vi "Preset_Manager_Main.vi"(4 "Virtual Devices List":string[](array[string]), 6 "Filtered Devices List":string[](array[string]), 8 "Experiment Name":string, 10 "DevStatusQueue":refnum<queue>, 11 "Software Root":string) -> ()   [LabVIEW 2020]
uses:
  Control 1.ctl
  <vilib>/Utility/miscctls.llb/LVRowAndColumnTypeDef.ctl
  Shared/MySQL/Preset Query Enum.ctl
  202ec612-3c63-4871-a0f5-fb571a4f3b4f.vi
  <vilib>/Array/Sort 2D Array - Pop Stack.vi
  <vilib>/Array/Sort 2D Array - Push Stack.vi
  <vilib>/Platform/browser.llb/Open URL in Default Browser (string).vi
  <vilib>/Utility/file.llb/Read Delimited Spreadsheet (string).vi
  <vilib>/Utility/file.llb/Write Delimited Spreadsheet (string).vi
  <userlib>/_OpenG.lib/array/array.llb/Delete Elements from 1D Array (String)__ogtk.vi
  <userlib>/_OpenG.lib/array/array.llb/Empty 1D Array (String)__ogtk.vi
  <vilib>/regexp/Match Regular Expression.xnode
panel:
  out "Queue Progress Bar":ext(slide) scale=0.0..1.0
  out "Queue Size":i32
  out "Current Preset Queue Element":string
  in  "Preset Devices Not On":i32(listbox)
  in  "Preset Devices Not in Experiment":i32(listbox)
  out "Active Preset":string
  out "Preset Execution Indicator":bool caption="Preset Aborted"
  in  "EXIT":bool
  in  "Using Queue":bool
  in  "Tab Control":T1(tab)
  in  "Dont jump \nto diagnostics":bool
  out "Currently Loaded":string
  in  "Reload Preset":bool caption="Reload"
  in  "Reload ECS":bool caption="Reload"
  in  "Preset Builder":bool
  in  "Execute Preset":bool
  in  "Delete Preset":bool
  in  "Save as Preset":bool
  in  "Preset Menu":u16(ring) items=["None", "2BL Amp2 16 J  Atte 100% BS 100T", "2BL Amp2 16 J Clunker IN 5% Attenuator", "2BL Amp2 16J Clunker OUT 5% att", "2BL Amp2 50/50", "2BL amp3 25 J 100T ", "2BL cameras triggered", "Amp 2 18 J 1BL", "Amp 3 25 J staging", "Amp2 Clunker In 1BL", "Amp2, MegaAttenuator", "Cameras free run - BELLA", "Cameras free run - DataLogging", "Cameras triggered - BELLA", "Cameras triggered - DataLogging", "Cameras triggered-1BL BELLA", "LT Amp1", "LT Amp2 17J", "LT Amp2 17J Clunker in", "LT Amp3 25 J Megaattenuator", "LT Amp3 25J", "LT Amp3 50J", "MagSpec TriggerOn", "MagSpecSimulateBoff", "MagSpecSimulateBon", "P2-WFS-LC", "SingleShot", "Stage 1 Cap in", "Stage 1 Cap out", "Stage 1 SMF in", "Stage 2 Gasjet IN", "Stage 2 Gasjet OUT", "Stage 2 SMF IN", "Stage 2 Tape Drive In and Aligned", "Stage 2 Tapedrive IN", "Stage 2 Tapedrive OUT", "Stage 2 YAG IN", "Staging APL In", "Staging APL out", "Z 1Hz", "Z Amp2 18 J", "Z Amp3 45 J 1BL Only", "Z Amp3 45 J OFI", "Z Amp3 45 J, Megaattenuator", "Z Diode obsolete", "Z amp2 , Clunker In", "Z amp2 12 J 80/20 OFI", "Z-Test-IN", "Z-Test22", "Z_TestPreset", "extra 2BL amp2 100T "]
  in  "Select an ECS file":path
  in  "Preset Table Control":string[][](table)
  in  "Choose Values":bool
  in  "Left Join":bool
  in  "Reset Queue":bool
  in  "Queue Table Control":string[][](table)
  in  "Queue Table":string[][](table)
  in  "Execute Queue":bool
  in  "Load Preset Queue":bool
  in  "Save Preset Queue":bool
  in  "Preset Queue Path":path
  out "Active Preset Achieved":bool
  out "Devices with Active \nPreset Not Set":string[](array[string])
  out "Dev Presets":string[](array[string])
  out "All Preset Devices ON?":bool[](array[boolean])
  in  "Abort Execution":T2
  in  "HELP WEB PAGE":bool
  out "PRESET FROM DB":string[][](table)
  out "ECS File":string[][](table)
  out "Coordinate Array":i32[][](array[numeric])
  out "Devices not started":string[](array[string]) caption="Devices not ready for scan"
  out "Active Device array":bool[](array[boolean])
  out "Active Dev/IP":string[](array[string])
  out "Device Errors":string[][](array[string])
  out "Queue Element":i32
  in  "Poll Count":i32
  out "error out":errorcluster
  out "Current State":string
  out "Remaining States":string
  # "Using CSV Files"
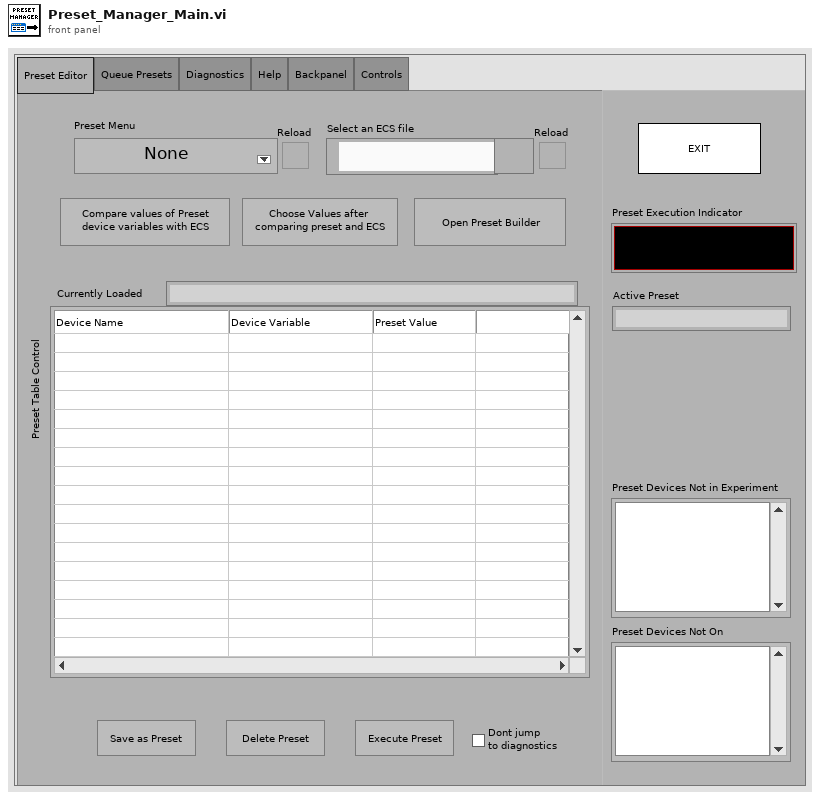
[diagram p1: front panel]
types:
  T1 = enum32{"Preset Editor", "Queue Presets", "Diagnostics", "Help", "Backpanel", "Controls"}
  T2 = typedef "Control 1.ctl" = bool
  T3 = typedef "LVRowAndColumnTypeDef.ctl" = cluster{"Row":i32, "Column":i32}
  T4 = typedef "Preset Query Enum.ctl" = enum16{"Get Locations", "Get all IPs and MACs", "Get classes", "Get expt variables to set at scanstart for particular device", "Get expt devices and variables with start values", "Get expt devices and variables (with data to get)", "Get expt devices with data to get", "Get Expt devices and GUIs", "Get all devices basic properties", "Get Virtual Devices Core Info", "Get Expt names", "Get experiment basic properties", "Get experiment alarm variables", "Get MC Ports", "Get device network comm port", "Get devicetype lvclass path", "Get basic device properties", "Get Init Order", "Get all setable variables of a device", "Get device variable aliases", "Get force values of all settable variables", "Get all variables of a devicetype", "Get all variables of a device", "Get plotter details", "Get Saved Scans", "Get Scan Info", "GetGeneralGUIs", "Get expt for plotter", "Get plotter IDs from expt", "Get all devices", "Get all Virtual Devices", "Get all aliases", "Get variable and device info for Virtual Device", "GetItemLocatorIP", "Get IPs for GUIs", "Get DeviceType from Device", "GetLocalPortRange", "GetDevicePresetVariables", "Get Device Configuration", "GetAllPresetNames", "GetAllConfigurationNames", "GetPresetDeviceNames", "GetDeviceAliases", "GetDevicesOfClass"}
  T5 = enum32{"Invalid", "Standard", "Closed", "Hidden", "Minimized", "Maximized"}
  T6 = enum32{"invalid app kind", "Development System", "Run Time System", "Student Edition", "Embedded LabVIEW", "Evaluation", "Custom"}
  T7 = cluster{"Core":cluster{"Current VI Reference":refnum<vi>, "Close Panel on Exit?":bool}, "Your Boolean data":bool, "String":string, "Preset Table Control":string[][], "Column Headers[]":string[], "Queue Table Control":string[][], "Preset Manager Cluster":cluster{"PresetName":string, "Mcast command":string, "Current Preset Devices":string[], "My IP":string, "Mcast address":string, "Software Root":string, "Experiment Name":string, "MCast Remote":u16, "UDP timeout ms":i32, "MC Multicast":refnum<k16>, "All Devices Core Info":string[][], "Filtered Devices List":string[], "Virtual Devices List":string[], "DevStatusQueue":refnum<queue>}, "Currently Loaded":string}
  T8 = typedef "LVPoint32TypeDef.ctl" = cluster{"Horizontal":i32, "Vertical":i32}
  T9 = cluster{"Current VI Reference":refnum<vi>, "Close Panel on Exit?":bool}
  T10 = cluster{"PresetName":string, "Mcast command":string, "Current Preset Devices":string[], "My IP":string, "Mcast address":string, "Software Root":string, "Experiment Name":string, "MCast Remote":u16, "UDP timeout ms":i32, "MC Multicast":refnum<k16>, "All Devices Core Info":string[][], "Filtered Devices List":string[], "Virtual Devices List":string[], "DevStatusQueue":refnum<queue>}
  T11 = enum16{"Left Button", "Center Button", "Right Button", "Window Close"}
  T12 = typedef "mysql_authentication.ctl" = cluster{"User":string, "Password":string, "Database":string}
  T13 = cluster{"Port":u16, "IP Address":string, "Authentication":T12}
  T14 = typedef "preset diagnostics.ctl" = cluster{"Active Preset Achieved":bool, "Devices with Active Preset Not Set":string[], "Dev Presets":string[], "All Preset Devices ON?":bool[]}
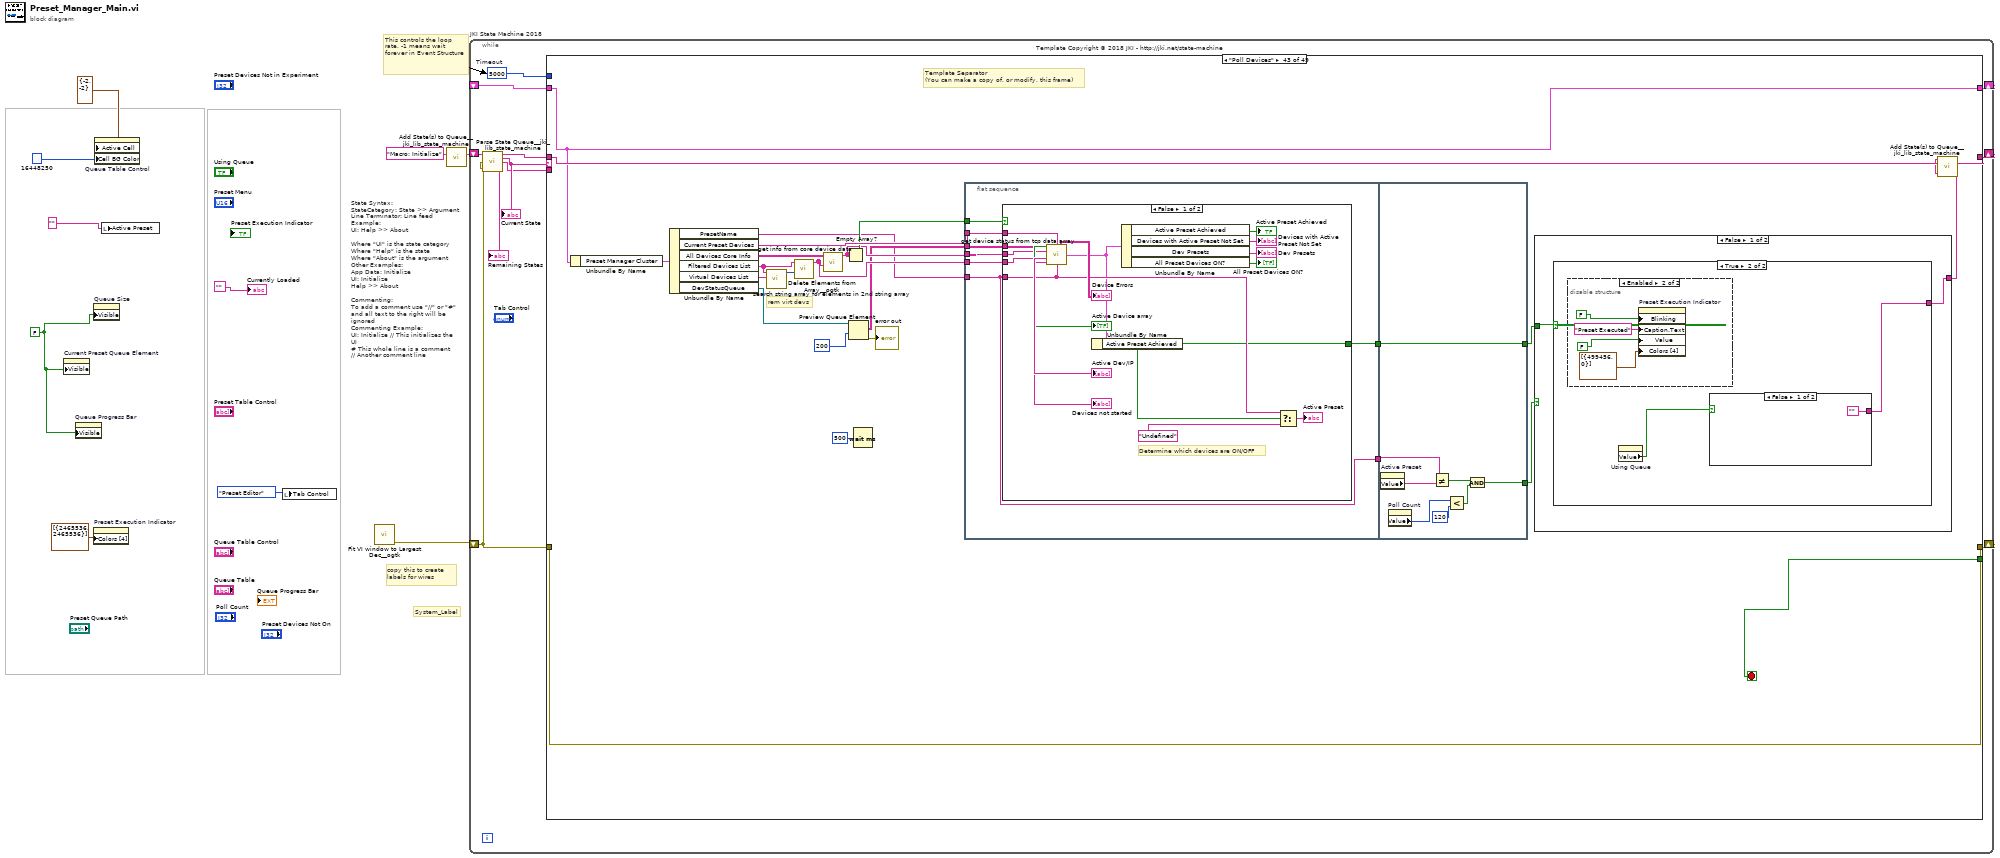
[diagram p0: block diagram]
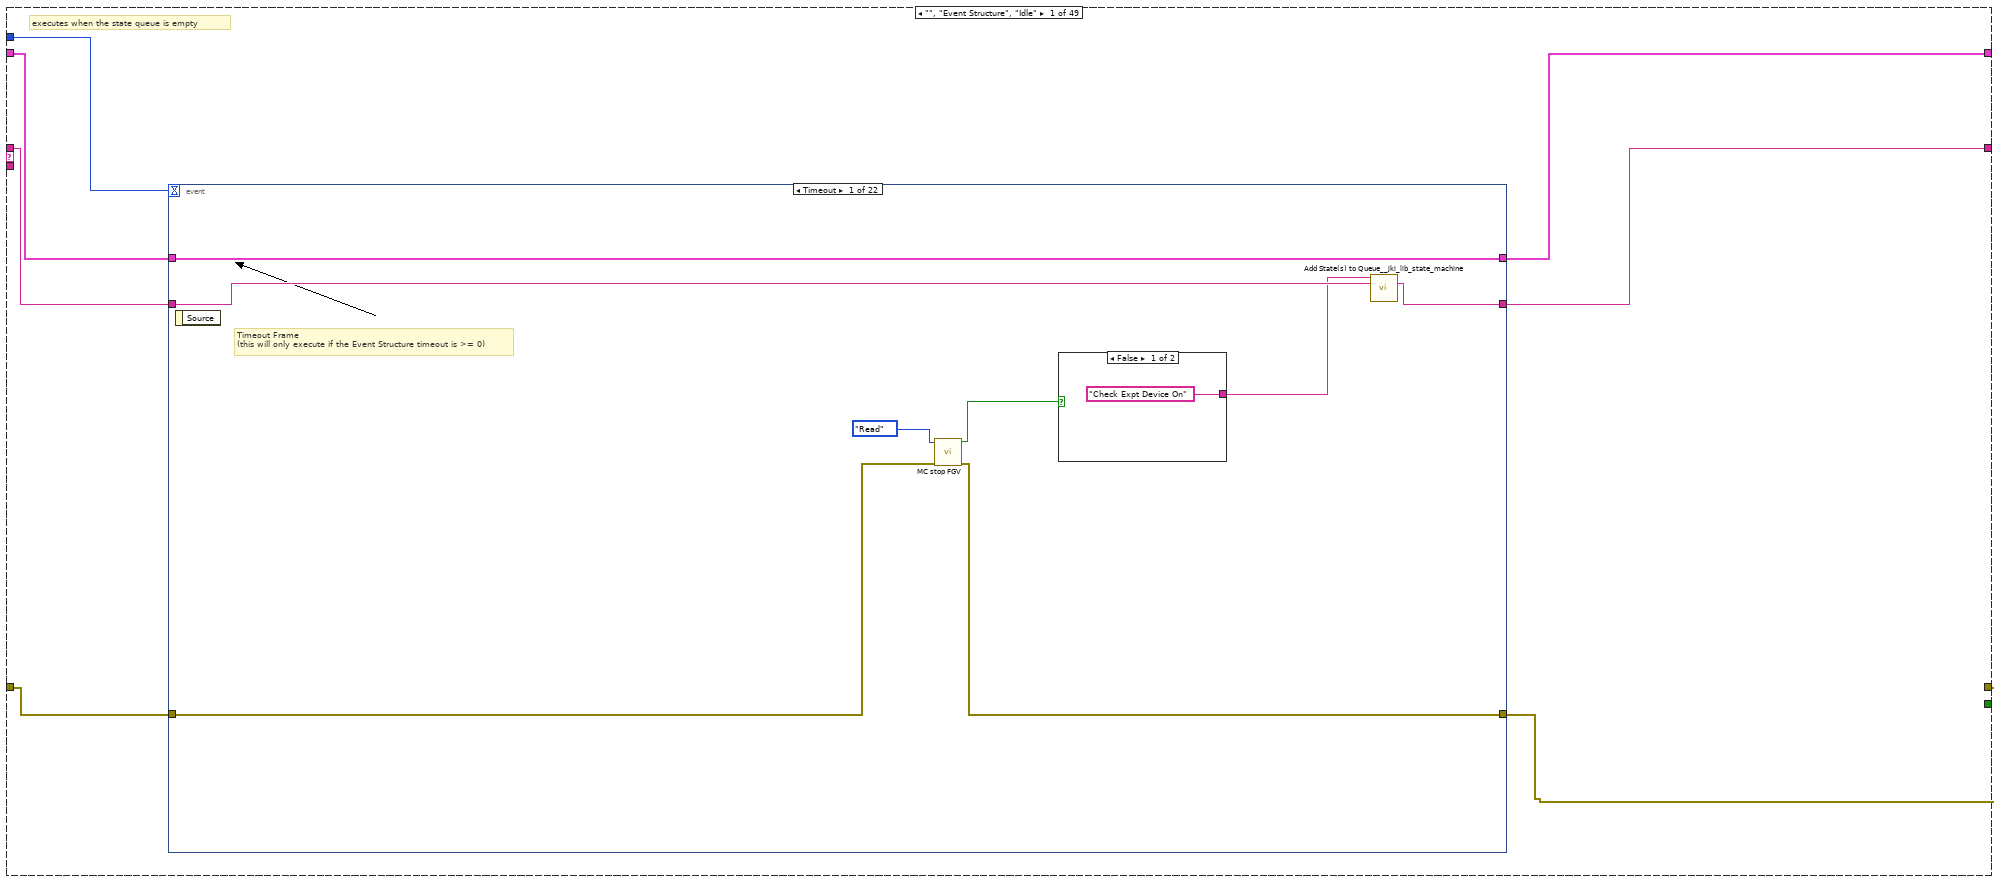
[diagram p2: hidden frame]
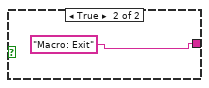
[diagram p3: hidden frame]
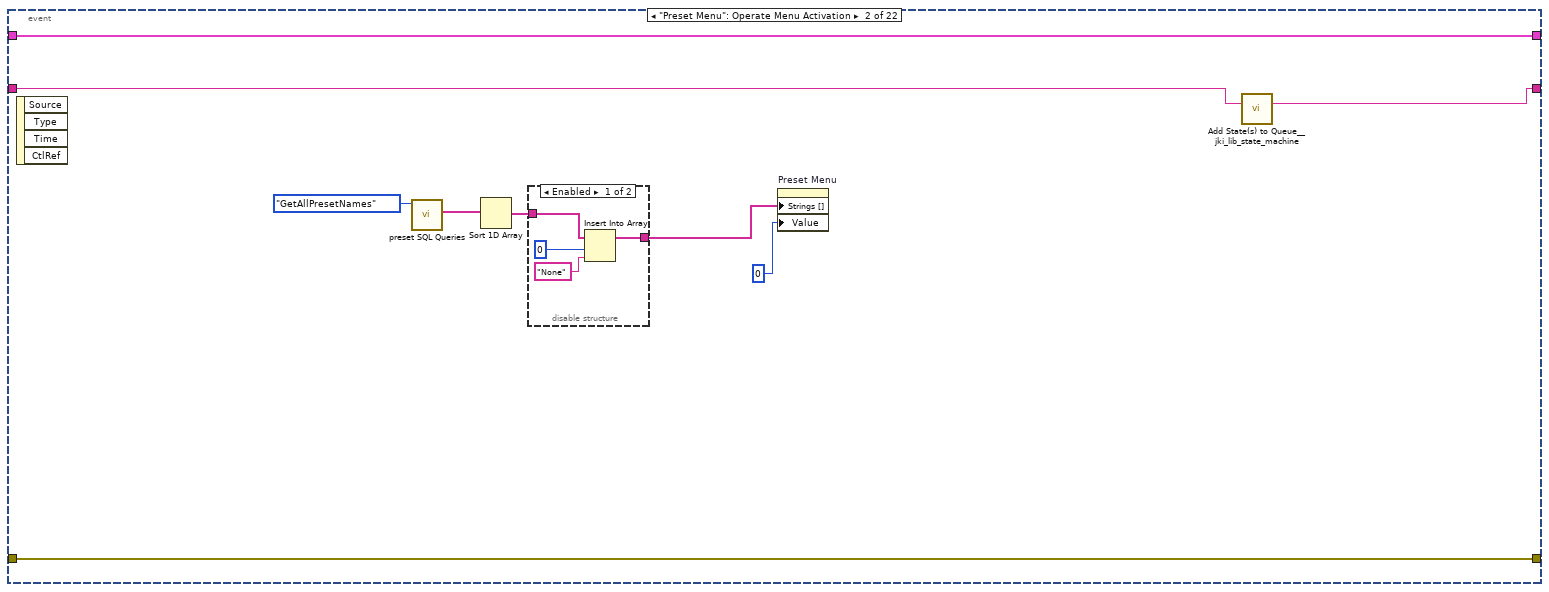
[diagram p4: hidden frame]
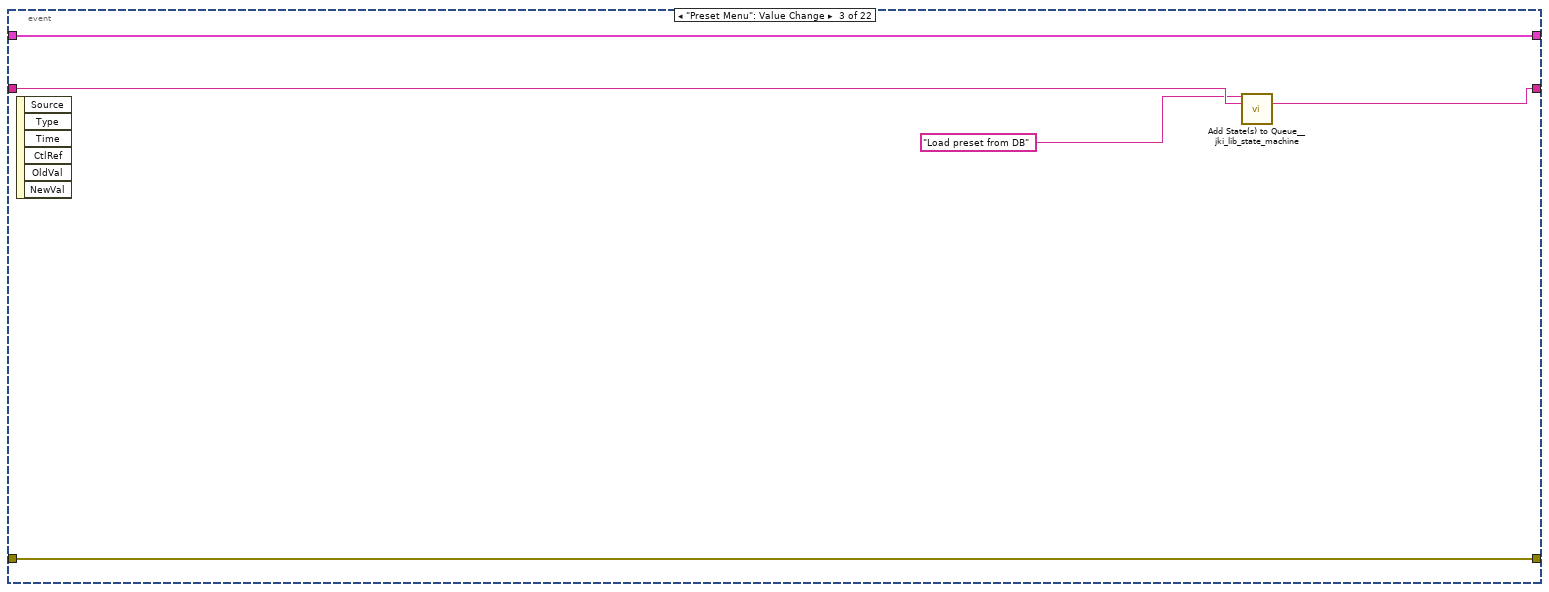
[diagram p6: hidden frame]
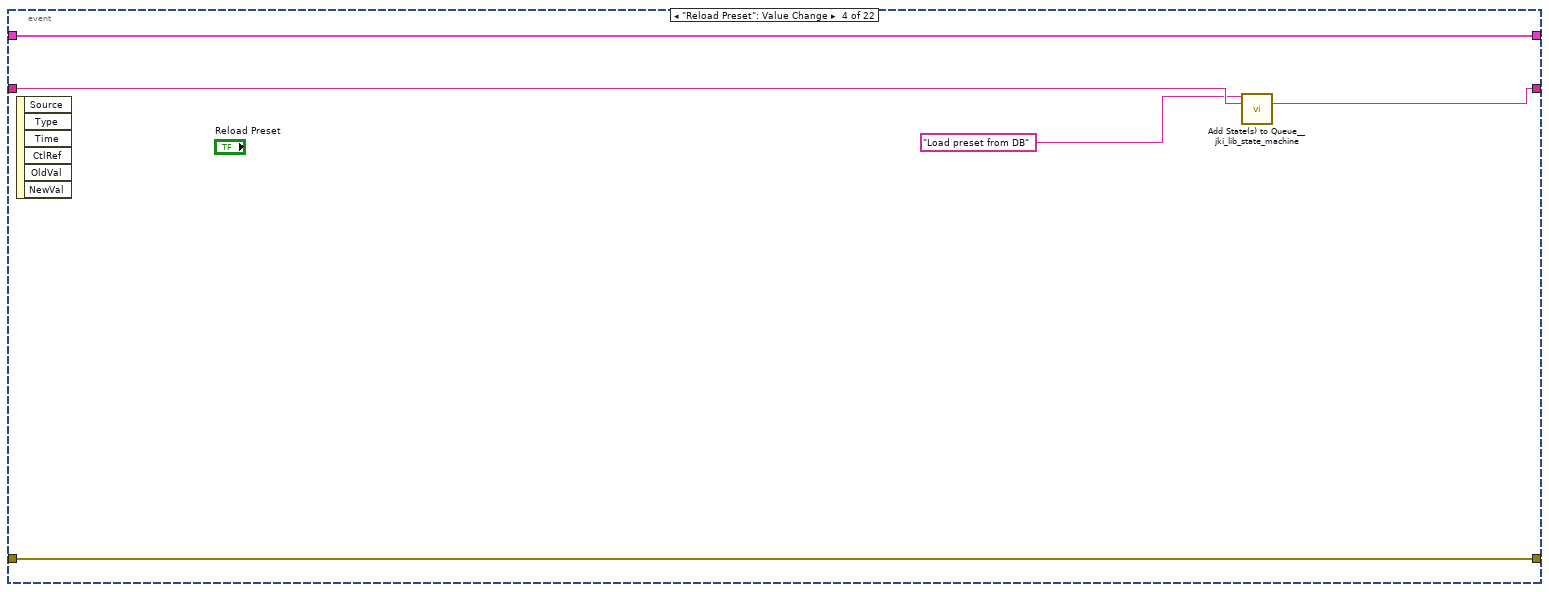
[diagram p7: hidden frame]
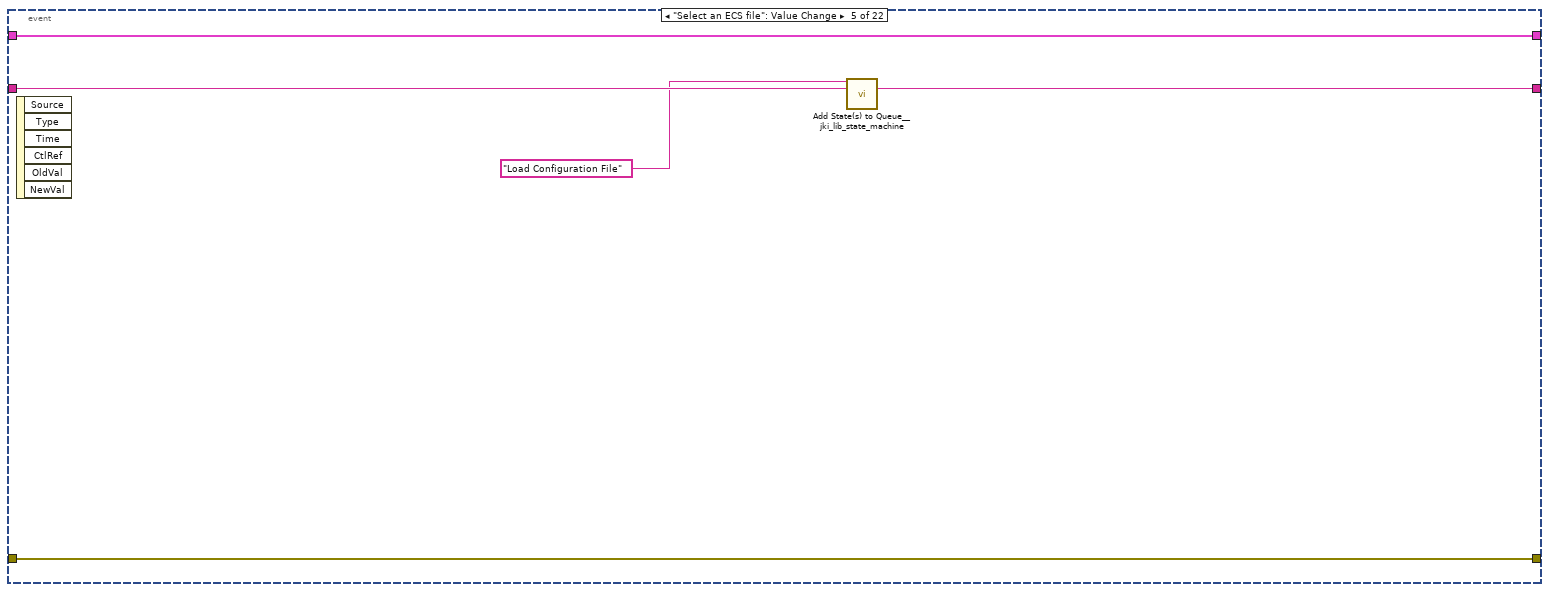
[diagram p8: hidden frame]
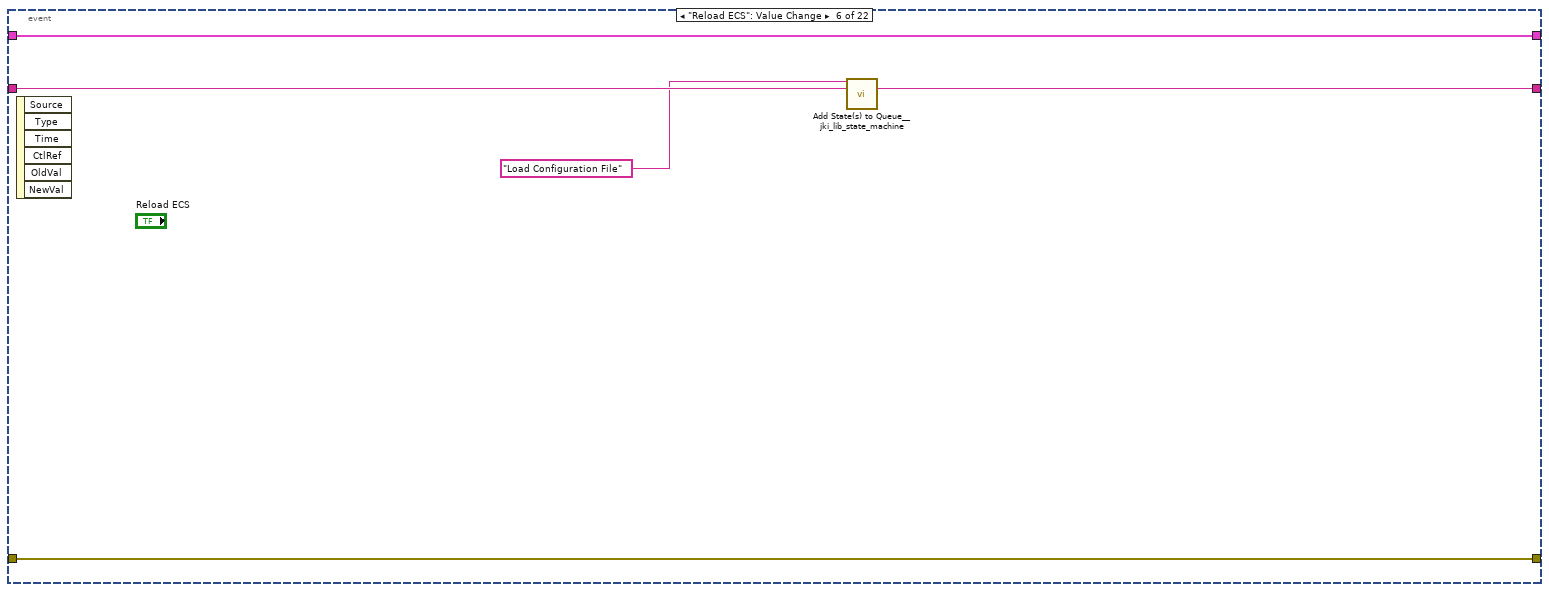
[diagram p9: hidden frame]
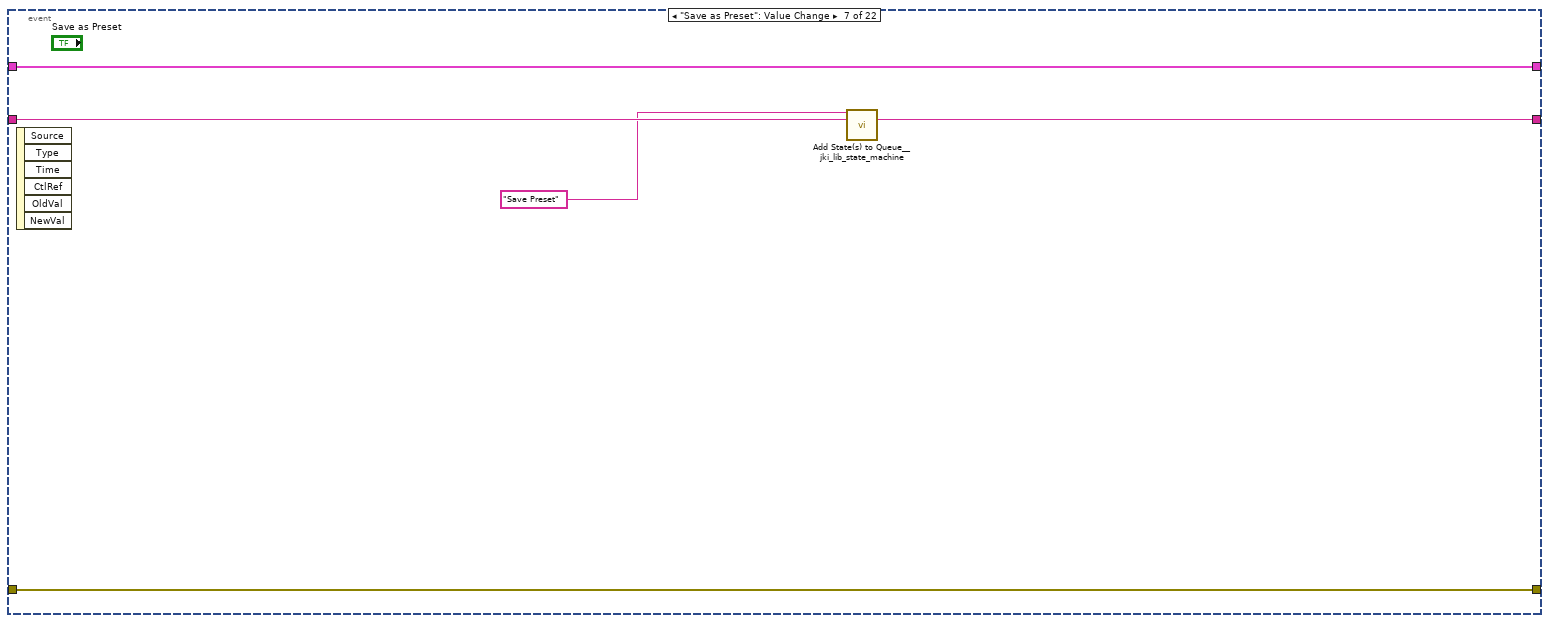
[diagram p10: hidden frame]
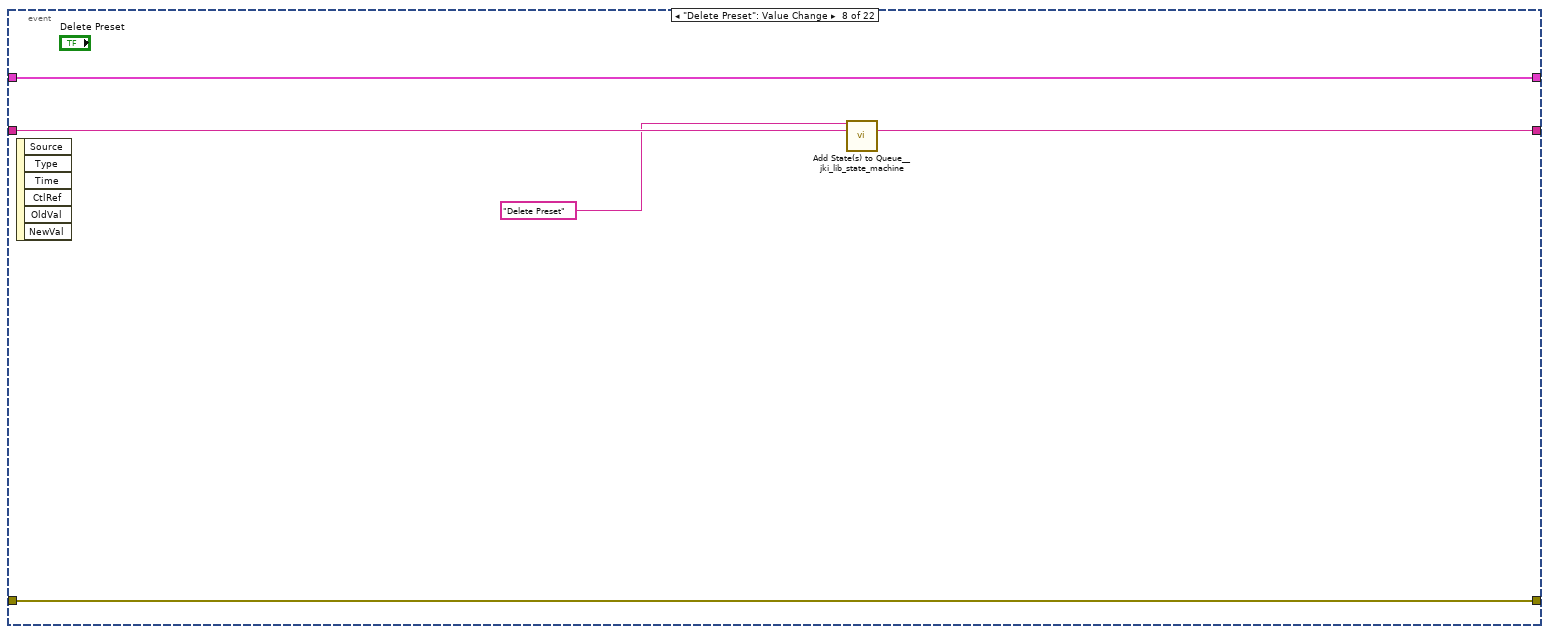
[diagram p11: hidden frame]
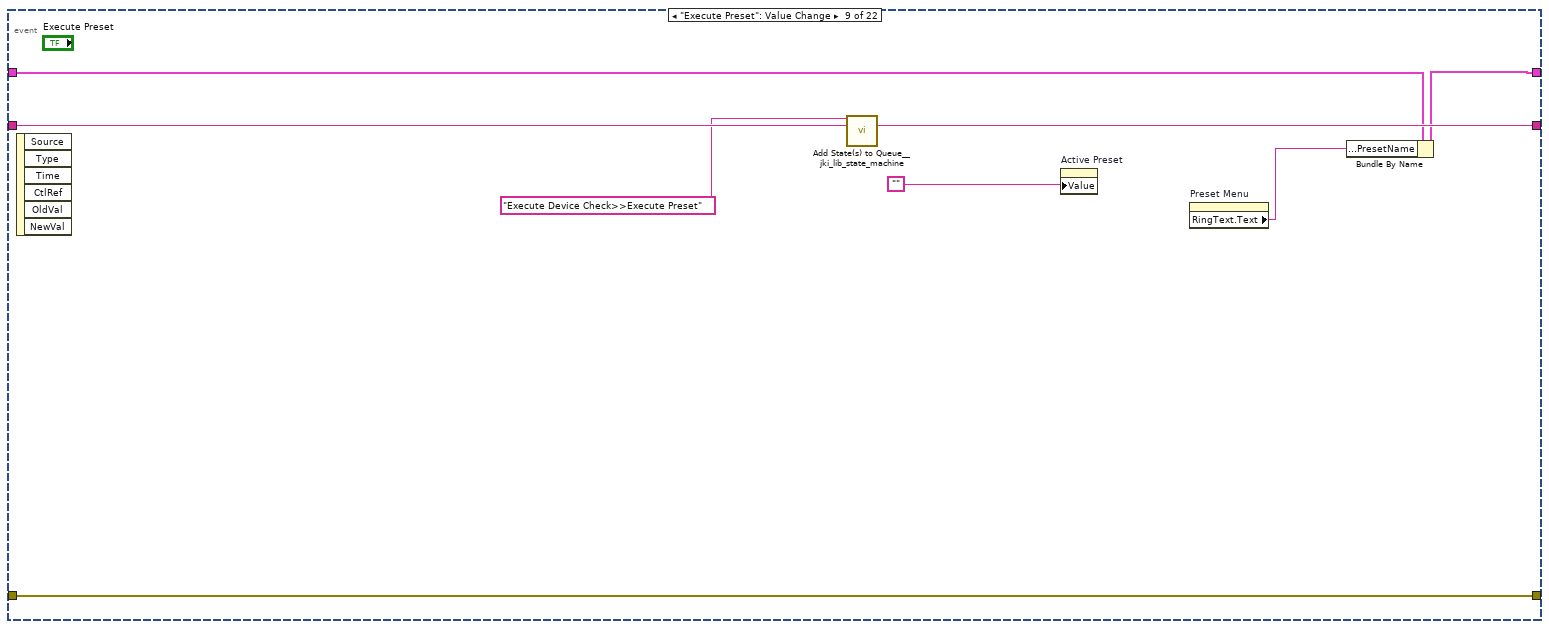
[diagram p12: hidden frame]
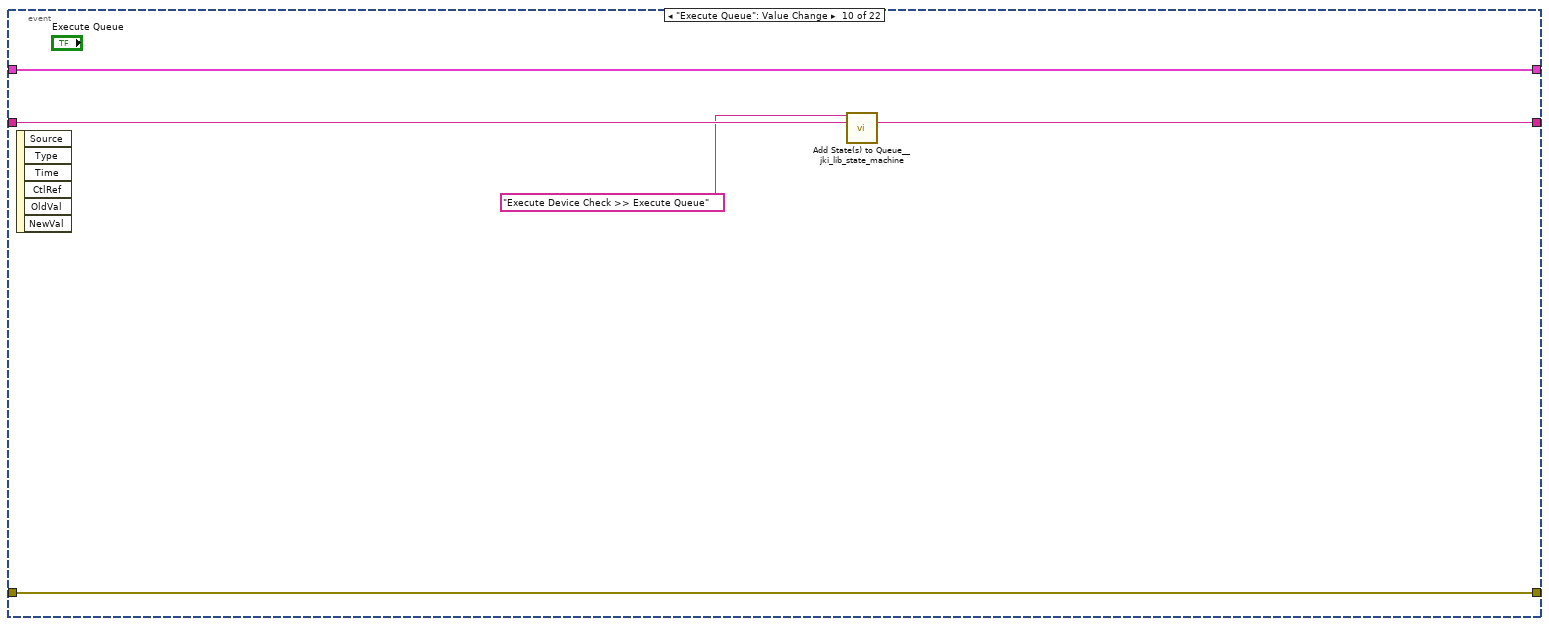
[diagram p13: hidden frame]
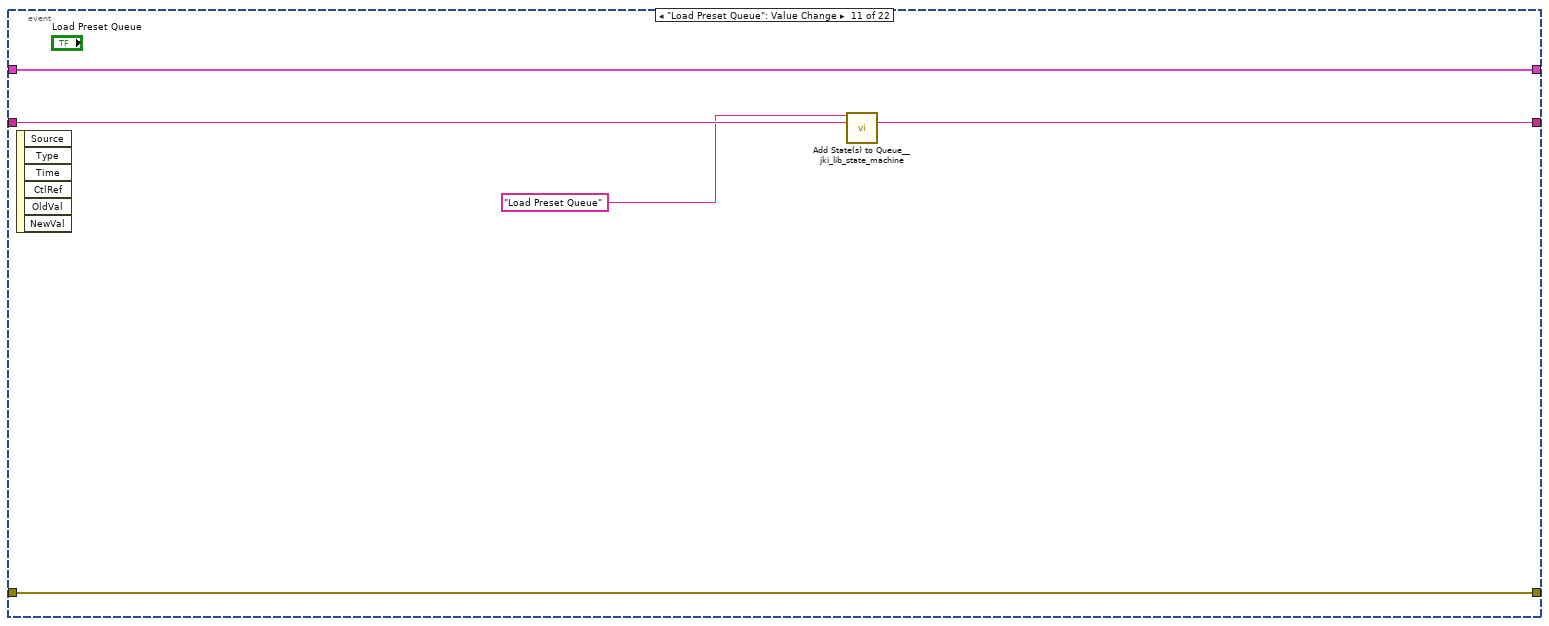
[diagram p14: hidden frame]
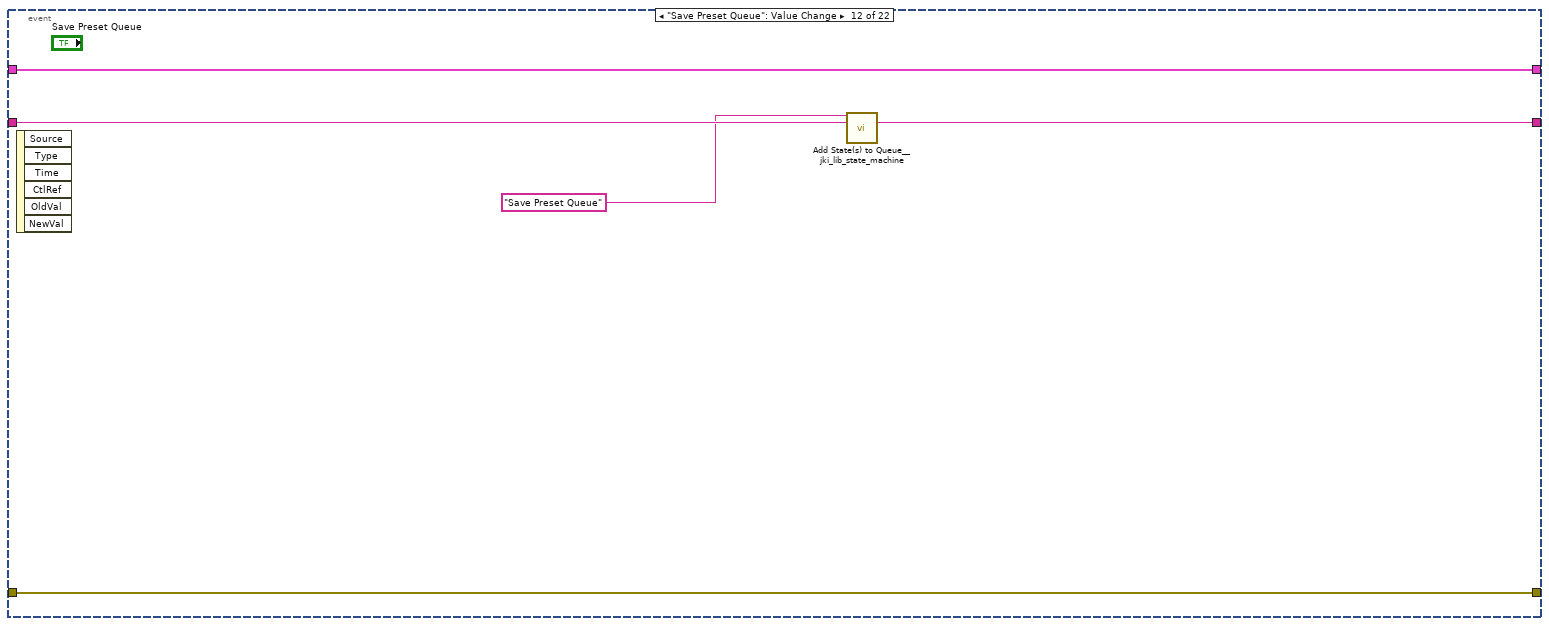
[diagram p15: hidden frame]
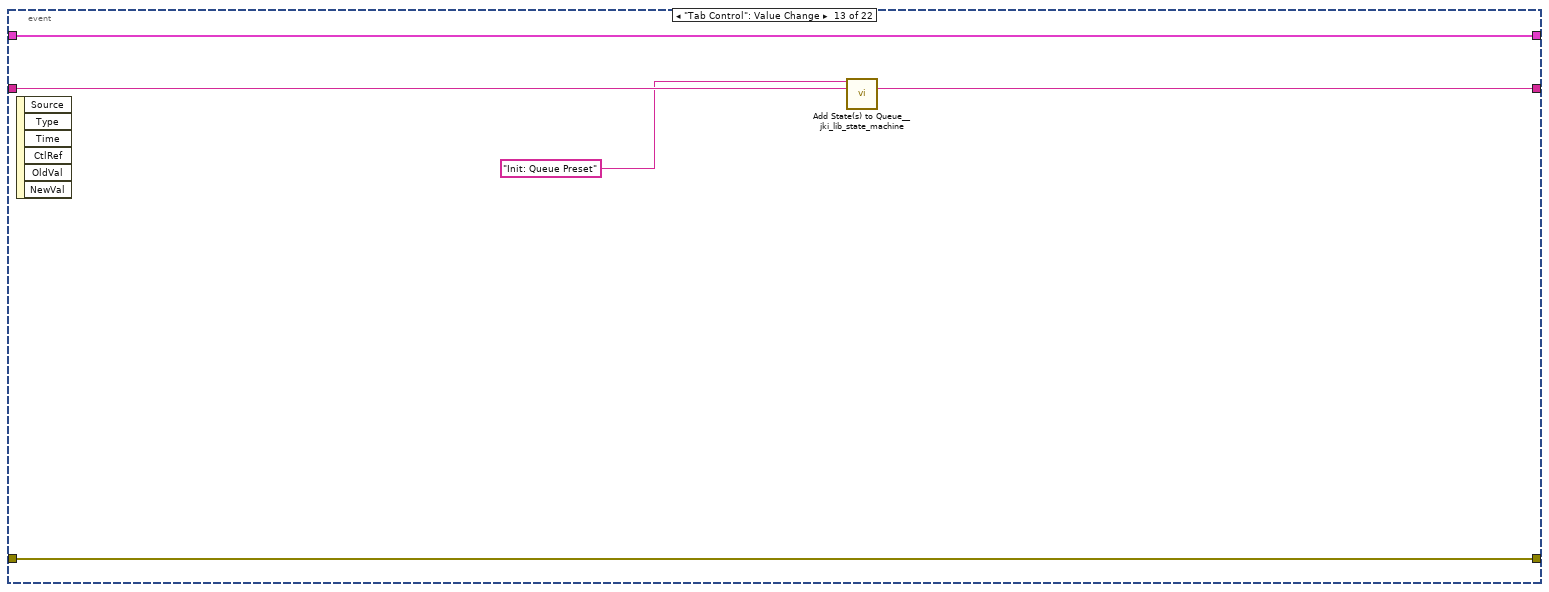
[diagram p16: hidden frame]
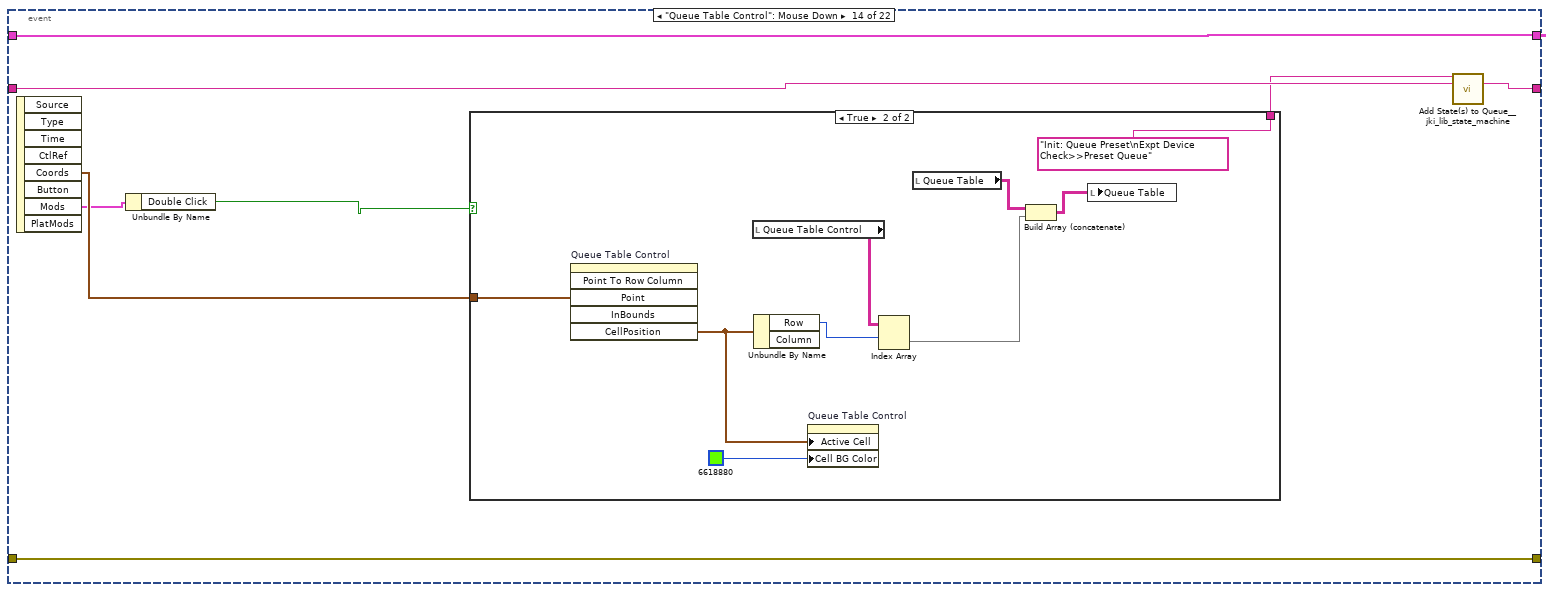
[diagram p17: hidden frame]
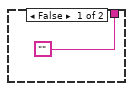
[diagram p18: hidden frame]
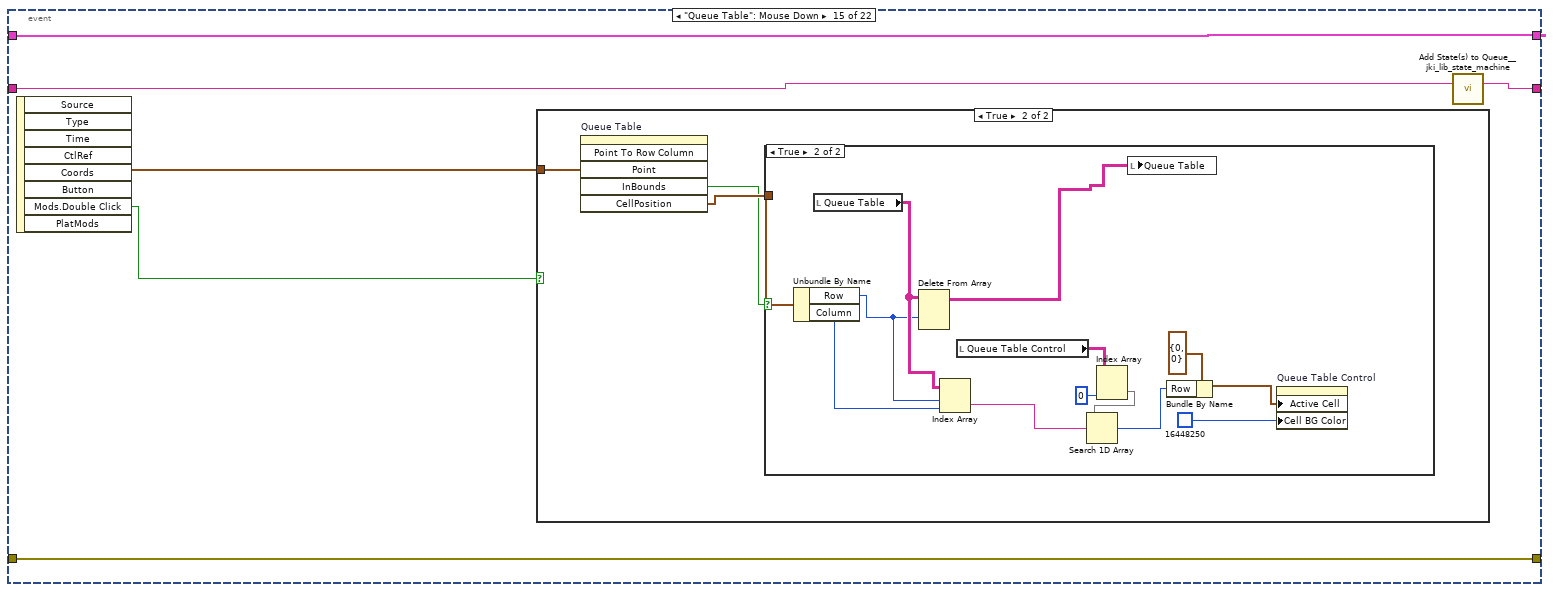
[diagram p19: hidden frame]
diagram:
  w5 = FALSE
  # "State Syntax:\nStateCategory: State >> Argument\nLine Terminator: Line feed\nExample:\nUI: Help >> About\n\nWhere \"UI\" is the state category\nWhere \"Help\" is the state\nWhere \"About\" is the argument\nOther Examples:\nApp Data: Initialize\nUI: Initialize\nHelp >> About\n\nCommenting:\nTo add a comment use \"//\" or \"#\" and all text to the right will be ignored\nCommenting Example:\nUI: Initialize // This initializes the UI\n# This whole line is a comment\n// Another comment line"
  # "copy this to create labels for wires"
  # "This controls the loop rate. -1 means wait forever in Event Structure"
  # "System_Label"
  n1 = property on="Current Preset Queue Element" class="Str"("Visible"=w5) -> ()  [unwired: 2 in, 2 out]
  n2 = property on="Queue Progress Bar" class="Slide (strict)"("Visible"=w5) -> ()  [unwired: 2 in, 2 out]
  n3 = property on="Queue Size" class="DigNum (strict)"("Visible"=w5) -> ()  [unwired: 2 in, 2 out]
  n4 = property on="Preset Execution Indicator" class="Bool (strict)"("Colors [4]"=cluster{u32, u32}[] [{2465536, 2465536}]) -> ()  [unwired: 2 in, 2 out]
  n5 = property on="Queue Table Control" class="Tbl (strict)"("Active Cell"=T3 {"Row"=-2, "Column"=-2} ("Active Cell:Active Cell"), "Cell BG Color"=u32 16448250 ("Active Cell:Cell Background Color")) -> ()  [unwired: 2 in, 2 out]
  n6 = local write "Active Preset"("" ("My IP")) -> ()
  n7 = local write "Tab Control"(T1."Preset Editor" ("Tab Control")) -> ()
  n8 = call <userlib>:"Fit VI window to Largest Dec__ogtk.vi"() -> ("error out"=w1:errorcluster)  [unwired: 6 in, 1 out]
  n9 = call <vilib>:"Add State(s) to Queue__jki_lib_state_machine.vi"("State(s) in (\"\")"="Macro: Initialize") -> ("States Out"=w10:string)  [unwired: 14 in]
  n10 = while "JKI State Machine 2018" {
    shift-right: [w11] -> _
    shift-left: _ -> [w14]
    shift-right: [w17] -> _
    shift-left: w1 -> [w12]
    shift-right: [w16] -> _
    shift-left: w10 -> [w18]
    stop <- w15 stop-if-true
    w13 = 5000  # Timeout
    # "Template Copyright © 2018 JKI - http://jki.net/state-machine"
    n11 = call <vilib>:"Parse State Queue__jki_lib_state_machine.vi"("State Queue"=w18, "Error In (no error)"=w12) -> ("Remaining States"=w20:string, "Current State"=w21:string, "Arguments"=w19:string)  [unwired: 11 in]
    "Current State" <- w21
    "Remaining States" <- w20
    n12 = case shown="\"Poll Devices\"" w21 {
      selector: w21 -> [_ _ w192 _ _ _ _ _ _ _ _ _ _ _ _ _ _ _ _ _ _ _ _ _ _ _ _ _ _ _ _ _ _ _ _ _ _ _ _ _ _ _ _ _ _ _ _ _ _]
      tunnel: w20 -> [w28 w191 w196 w215 w221 w226 w230 w248 w254 w258 w262 w268 w279 w348 w361 w371 w383 w396 w400 w414 w422 w432 w444 w453 w467 w593 w610 w636 w670 w687 w692 w698 w702 w708 w714 w721 w733 w739 w754 w781 w788 w794 w825 w896 w912 w916 w922 w947 w982]
      tunnel: w19 -> [_ _ _ _ _ _ _ _ _ _ _ w263 w273 _ _ _ _ _ _ _ _ _ _ _ _ _ _ _ _ _ _ _ _ _ _ _ _ _ _ _ w782 _ _ _ w901 _ w918 w943 _]
      tunnel: w14 -> [w26 w188 w194 w208 w218 w224 w227 _ w249 w255 w260 w266 w275 w345 w358 w368 w380 w392 w397 w405 w415 w428 w440 w450 w464 w582 w607 w633 w666 w684 w689 w695 w699 w703 w712 w716 w730 w736 w750 w778 w785 w791 w821 w889 w904 w913 w919 w944 w979]
      tunnel: [w25 w189 w198 w212 errorcluster {"status"=FALSE, "code"=0, "source"=""} ("error out") w223 w228 w246 w250 w256 w259 w264 w276 w346 w359 w369 w381 w394 w398 w412 w420 w430 w442 w451 w465 w591 w608 w634 w668 w685 w690 w696 w700 w705 w710 w719 w731 w737 w752 w779 w786 w792 w823 w894 w910 w914 w920 w945 w980] -> w17
      tunnel: w12 -> [w24 w189 w197 w212 w217 w223 w228 w246 w251 w256 w259 w265 w277 w346 w359 w369 w381 w394 w398 w412 w420 w430 w442 w451 w465 w591 w608 w634 w668 w685 w690 w696 w700 w706 w711 w719 w731 w737 w752 w779 w786 w792 w823 w894 w910 w914 w920 w945 w980]
      tunnel: [w27 w190 w195 w214 w220 w225 w229 w247 w253 w257 w261 w267 w278 w347 w360 w370 w382 w395 w399 w413 w421 w431 w443 w452 w466 w592 w609 w635 w669 w686 w691 w697 w701 w707 w713 w720 w732 w738 w753 w780 w787 w793 w824 w895 w911 w915 w921 w946 w981] -> w16
      tunnel: [_ _ _ _ _ TRUE _ _ _ _ _ _ _ _ _ _ _ _ _ _ _ _ _ _ _ _ _ _ _ _ _ _ _ _ _ _ _ _ _ _ _ _ _ _ _ _ _ _ _] -> w15
      tunnel: w13 -> [w22 _ _ _ _ _ _ _ _ _ _ _ _ _ _ _ _ _ _ _ _ _ _ _ _ _ _ _ _ _ _ _ _ _ _ _ _ _ _ _ _ _ _ _ _ _ _ _ _]
      tunnel: [w23 w188 w194 w213 w218 w224 w227 w237 w249 w255 w260 w266 w275 w345 w358 w368 w379 w392 w397 w408 w415 w427 w439 w449 w463 w582 w607 w633 w666 w684 w689 w695 w699 w703 w712 w716 w730 w736 w749 w778 w785 w791 w821 w890 w903 w913 w919 w944 w979] -> w11
      frame "", "Event Structure", "Idle" {
        # "executes when the state queue is empty"
        n13 = event shown="[0] Timeout" {
          selector: _ -> [_ _ _ _ _ _ _ _ _ _ _ _ _ _ _ _ _ _ _ _ _ _]
          dyn-events: _ -> [_ _ _ _ _ _ _ _ _ _ _ _ _ _ _ _ _ _ _ _ _ _]
          timeout: w22 -> [_ _ _ _ _ _ _ _ _ _ _ _ _ _ _ _ _ _ _ _ _ _]
          tunnel: w28 -> [w36 w43 w55 w60 w65 w70 w75 w80 w89 w93 w98 w103 w109 w117 w133 w153 w158 w163 w168 w173 w180 w187]
          tunnel: [w35 w42 w54 w59 w64 w69 w74 w79 w88 w92 w97 w102 w108 w116 w132 w152 w157 w162 w167 w172 w179 w186] -> w27
          tunnel: w26 -> [w34 w47 w57 w62 w67 w72 w77 w82 w84 w95 w100 w105 w106 w114 w131 w155 w160 w165 w170 w175 w177 w184]
          tunnel: [w30 w46 w56 w61 w66 w71 w76 w81 w90 w94 w99 w104 w110 w118 w134 w154 w159 w164 w169 w174 w178 w185] -> w25
          tunnel: w24 -> [w31 w46 w56 w61 w66 w71 w76 w81 w90 w94 w99 w104 w110 w118 w134 w154 w159 w164 w169 w174 w178 w185]
          tunnel: [w34 w47 w57 w62 w67 w72 w77 w82 w83 w95 w100 w105 w106 w114 w131 w155 w160 w165 w170 w175 w177 w184] -> w23
          event Timeout {
            # "Timeout Frame\n(this will only execute if the Event Structure timeout is >= 0)"
            n14 = event-data() -> ()  [unwired: 1 in, 1 out]
            n15 = call "MC stop FGV.vi"("error in"=w31, "Function"=enum16{"Read", "Write", "Clear"}."Read") -> ("error out"=w30:errorcluster, "Stop out"=w29:bool)  [unwired: 8 in]
            n16 = case shown="False" w29 {
              tunnel: ["Check Expt Device On" ("State(s) in Front (\"\")") "Macro: Exit"] -> w33
              frame False {
              }
              frame True {
              }
            }
            n17 = call <vilib>:"Add State(s) to Queue__jki_lib_state_machine.vi"("State(s) in Front (\"\")"=w33, "State(s) in (\"\")"=w36) -> ("States Out"=w35:string)  [unwired: 13 in]
          }
          event "Preset Menu": Operate Menu Activation {
            n18 = event-data() -> ()  [unwired: 1 in, 4 out]
            n19 = call "preset SQL Queries.vi"("Preset Query"=Preset_Query_Enum."GetAllPresetNames") -> ("1st column 1st data"=w41:string[])  [unwired: 8 in, 2 out]
            n20 = Sort 1D Array(array=w41) -> (sorted array=w40:string[])
            n21 = disable-structure shown="Enabled" {
              disable-tunnel: w40 -> [w49 w52]
              disable-tunnel: [w48 w52] -> w39
              frame Enabled {
                n22 = Insert Into Array(array=w49, index=0, new element="None" ("new element/subarray")) -> (w48:string[])
              }
              frame Disabled {
              }
            }
            n23 = property on="Preset Menu" class="Ring (strict)"("Strings []"=w39, "Value"=0 ("index")) -> ()  [unwired: 2 in, 2 out]
            n24 = call <vilib>:"Add State(s) to Queue__jki_lib_state_machine.vi"("State(s) in (\"\")"=w43) -> ("States Out"=w42:string)  [unwired: 14 in]
          }
          event "Preset Menu": Value Change {
            n25 = event-data() -> ()  [unwired: 1 in, 6 out]
            n26 = call <vilib>:"Add State(s) to Queue__jki_lib_state_machine.vi"("State(s) in Front (\"\")"="Load preset from DB" ("State(s) in Front (\"\")"), "State(s) in (\"\")"=w55) -> ("States Out"=w54:string)  [unwired: 13 in]
          }
          event "Reload Preset": Value Change {
            n27 = event-data() -> ()  [unwired: 1 in, 6 out]
            n28 = call <vilib>:"Add State(s) to Queue__jki_lib_state_machine.vi"("State(s) in Front (\"\")"="Load preset from DB" ("State(s) in Front (\"\")"), "State(s) in (\"\")"=w60) -> ("States Out"=w59:string)  [unwired: 13 in]
          }
          event "Select an ECS file": Value Change {
            n29 = event-data() -> ()  [unwired: 1 in, 6 out]
            n30 = call <vilib>:"Add State(s) to Queue__jki_lib_state_machine.vi"("State(s) in Front (\"\")"="Load Configuration File", "State(s) in (\"\")"=w65) -> ("States Out"=w64:string)  [unwired: 13 in]
          }
          event "Reload ECS": Value Change {
            n31 = event-data() -> ()  [unwired: 1 in, 6 out]
            n32 = call <vilib>:"Add State(s) to Queue__jki_lib_state_machine.vi"("State(s) in Front (\"\")"="Load Configuration File", "State(s) in (\"\")"=w70) -> ("States Out"=w69:string)  [unwired: 13 in]
          }
          event "Save as Preset": Value Change {
            n33 = event-data() -> ()  [unwired: 1 in, 6 out]
            n34 = call <vilib>:"Add State(s) to Queue__jki_lib_state_machine.vi"("State(s) in Front (\"\")"="Save Preset", "State(s) in (\"\")"=w75) -> ("States Out"=w74:string)  [unwired: 13 in]
          }
          event "Delete Preset": Value Change {
            n35 = event-data() -> ()  [unwired: 1 in, 6 out]
            n36 = call <vilib>:"Add State(s) to Queue__jki_lib_state_machine.vi"("State(s) in Front (\"\")"="Delete Preset", "State(s) in (\"\")"=w80) -> ("States Out"=w79:string)  [unwired: 13 in]
          }
          event "Execute Preset": Value Change {
            n37 = event-data() -> ()  [unwired: 1 in, 6 out]
            n38 = call <vilib>:"Add State(s) to Queue__jki_lib_state_machine.vi"("State(s) in Front (\"\")"="Execute Device Check>>Execute Preset", "State(s) in (\"\")"=w89) -> ("States Out"=w88:string)  [unwired: 13 in]
            n39 = property on="Active Preset" class="Str"("Value"="") -> ()  [unwired: 2 in, 2 out]
            n40 = property on="Preset Menu" class="Ring (strict)"() -> ("RingText.Text"=w85:string)  [unwired: 2 in, 2 out]
            n41 = Bundle By Name(cluster=w84, "Preset Manager Cluster.PresetName"=w85) -> (w83:T7)
          }
          event "Execute Queue": Value Change {
            n42 = event-data() -> ()  [unwired: 1 in, 6 out]
            n43 = call <vilib>:"Add State(s) to Queue__jki_lib_state_machine.vi"("State(s) in Front (\"\")"="Execute Device Check >> Execute Queue", "State(s) in (\"\")"=w93) -> ("States Out"=w92:string)  [unwired: 13 in]
          }
          event "Load Preset Queue": Value Change {
            n44 = event-data() -> ()  [unwired: 1 in, 6 out]
            n45 = call <vilib>:"Add State(s) to Queue__jki_lib_state_machine.vi"("State(s) in Front (\"\")"="Load Preset Queue", "State(s) in (\"\")"=w98) -> ("States Out"=w97:string)  [unwired: 13 in]
          }
          event "Save Preset Queue": Value Change {
            n46 = event-data() -> ()  [unwired: 1 in, 6 out]
            n47 = call <vilib>:"Add State(s) to Queue__jki_lib_state_machine.vi"("State(s) in Front (\"\")"="Save Preset Queue", "State(s) in (\"\")"=w103) -> ("States Out"=w102:string)  [unwired: 13 in]
          }
          event "Tab Control": Value Change {
            n48 = event-data() -> ()  [unwired: 1 in, 6 out]
            n49 = call <vilib>:"Add State(s) to Queue__jki_lib_state_machine.vi"("State(s) in Front (\"\")"="Init: Queue Preset", "State(s) in (\"\")"=w109) -> ("States Out"=w108:string)  [unwired: 13 in]
          }
          event "Queue Table Control": Mouse Down {
            n50 = event-data() -> ("Coords"=w113:T8, "Mods"=w112:cluster{"Double Click":bool, "Menu Key":bool})  [unwired: 1 in, 6 out]
            n51 = Unbundle By Name(w112) -> ("Double Click"=w111:bool)
            n52 = case shown="True" w111 {
              tunnel: ["" "Init: Queue Preset\nExpt Device Check>>Preset Queue"] -> w115
              tunnel: w113 -> [_ w127]
              frame False {
              }
              frame True {
                n53 = invoke on="Queue Table Control" class="Tbl (strict)" method="Point To Row Column"("Point"=w127) -> ("CellPosition"=w124:T3)  [unwired: 5 in, 5 out]
                n54 = local read "Queue Table Control"() -> (w126:string[][])
                n55 = Unbundle By Name(w124) -> ("Row"=w125:i32)  [unwired: 1 out]
                n56 = property on="Queue Table Control" class="Tbl (strict)"("Active Cell"=w124, "Cell BG Color"=u32 6618880 ("Active Cell:Cell Background Color")) -> ()  [unwired: 2 in, 2 out]
                n57 = Index Array(array=w126, index (row)=w125) -> (element=w122:string[])  [unwired: 1 in]
                n58 = local read "Queue Table"() -> (w120:string[][])
                n59 = Build Array (concatenate)(w120, w122) -> (w121:string[][])
                n60 = local write "Queue Table"(w121) -> ()
              }
            }
            n61 = call <vilib>:"Add State(s) to Queue__jki_lib_state_machine.vi"("State(s) in Front (\"\")"=w115, "State(s) in (\"\")"=w117) -> ("States Out"=w116:string)  [unwired: 13 in]
          }
          event "Queue Table": Mouse Down {
            n62 = event-data() -> ("Coords"=w130:T8, "Mods.Double Click"=w129:bool)  [unwired: 1 in, 6 out]
            n63 = case shown="True" w129 {
              tunnel: w130 -> [_ w137]
              frame False {
              }
              frame True {
                n64 = invoke on="Queue Table" class="Tbl (strict)" method="Point To Row Column"("Point"=w137) -> ("InBounds"=w135:bool, "CellPosition"=w136:T3)  [unwired: 5 in, 4 out]
                n65 = case shown="True" w135 {
                  tunnel: w136 -> [_ w150]
                  frame False {
                  }
                  frame True {
                    n66 = Unbundle By Name(w150) -> ("Row"=w147:i32, "Column"=w146:i32)
                    n67 = local read "Queue Table"() -> (w148:string[][])
                    n68 = Delete From Array(array=w148, index (row)=w147) -> (array with subset deleted=w149:string[][])  [unwired: 2 in, 1 out]
                    n69 = Index Array(array=w148, index (row)=w147, index (col)=w146) -> (element=w145:string)
                    n70 = local read "Queue Table Control"() -> (w144:string[][])
                    n71 = Index Array(array=w144, index (col)=0 ("disabled index (col)")) -> (element=w142:string[])  [unwired: 1 in]
                    n72 = Search 1D Array(1D array=w142, element=w145) -> (index of element=w138:i32)  [unwired: 1 in]
                    n73 = local write "Queue Table"(w149) -> ()
                    n74 = Bundle By Name(cluster=T3 {"Row"=0, "Column"=0} ("Active Cell:Active Cell"), "Row"=w138) -> (w139:T3)
                    n75 = property on="Queue Table Control" class="Tbl (strict)"("Active Cell"=w139, "Cell BG Color"=u32 16448250 ("Active Cell:Cell Background Color")) -> ()  [unwired: 2 in, 2 out]
                  }
                }
              }
            }
            n76 = call <vilib>:"Add State(s) to Queue__jki_lib_state_machine.vi"("State(s) in (\"\")"=w133) -> ("States Out"=w132:string)  [unwired: 14 in]
          }
          event "Left Join": Value Change {
            n77 = event-data() -> ()  [unwired: 1 in, 6 out]
            n78 = call <vilib>:"Add State(s) to Queue__jki_lib_state_machine.vi"("State(s) in Front (\"\")"="Compare Table", "State(s) in (\"\")"=w153) -> ("States Out"=w152:string)  [unwired: 13 in]
          }
          event "HELP WEB PAGE": Value Change {
            n79 = event-data() -> ()  [unwired: 1 in, 6 out]
            n80 = call-poly <vilib>:"Open URL in Default Browser.vi"("URL"="https://sites.google.com/a/lbl.gov/geecs/preset-manager?authuser=0") -> ()  [unwired: 5 in, 2 out]
            n81 = call <vilib>:"Add State(s) to Queue__jki_lib_state_machine.vi"("State(s) in (\"\")"=w158) -> ("States Out"=w157:string)  [unwired: 14 in]
          }
          event "Preset Builder": Value Change {
            n82 = event-data() -> ()  [unwired: 1 in, 6 out]
            n83 = call <vilib>:"Add State(s) to Queue__jki_lib_state_machine.vi"("State(s) in Front (\"\")"="Preset Builder" ("State(s) in Front (\"\")"), "State(s) in (\"\")"=w163) -> ("States Out"=w162:string)  [unwired: 13 in]
          }
          event "Reset Queue": Value Change {
            n84 = event-data() -> ()  [unwired: 1 in, 6 out]
            n85 = call <vilib>:"Add State(s) to Queue__jki_lib_state_machine.vi"("State(s) in Front (\"\")"="Reset Queue", "State(s) in (\"\")"=w168) -> ("States Out"=w167:string)  [unwired: 13 in]
          }
          event "Choose Values": Value Change {
            (unwired) FALSE ("Choose Values")
            n86 = event-data() -> ()  [unwired: 1 in, 6 out]
            n87 = call <vilib>:"Add State(s) to Queue__jki_lib_state_machine.vi"("State(s) in Front (\"\")"="Compare Table\nChoose Values", "State(s) in (\"\")"=w173) -> ("States Out"=w172:string)  [unwired: 13 in]
          }
          event "EXIT": Value Change {
            # "Exit Button Value Change (pressed) Event\n(this executes Macro: Exit to terminate the VI)"
            n88 = event-data() -> ()  [unwired: 1 in, 1 out]
            n89 = call <vilib>:"Add State(s) to Queue__jki_lib_state_machine.vi"("State(s) in Front (\"\")"="Macro: Exit", "State(s) in (\"\")"=w180) -> ("States Out"=w179:string)  [unwired: 13 in]
          }
          event Panel Close? {
            # "Discard the event because we'll close the front panel ourselves in Macro: Exit"
            # "Close Panel button (pressed) Event\n(this executes Macro: Exit to terminate the VI)"
            n90 = event-data() -> ()  [unwired: 1 in, 1 out]
            n91 = local write "Abort Execution"(T2 TRUE ("Abort Execution")) -> ()
            n92 = call <vilib>:"Add State(s) to Queue__jki_lib_state_machine.vi"("State(s) in Front (\"\")"="Check Abort\nMacro: Exit", "State(s) in (\"\")"=w187) -> ("States Out"=w186:string)  [unwired: 13 in]
            n93 = event-data("Discard?"=TRUE) -> ()  [unwired: 1 in, 1 out]
          }
        }
      }
      frame "---------- Core ----------" {
        # "Do not put any code in this frame.\n(it is a separator no-op)"
        n94 = call <vilib>:"Add State(s) to Queue__jki_lib_state_machine.vi"("State(s) in (\"\")"=w191) -> ("States Out"=w190:string)  [unwired: 14 in]
      }
      frame Default {
        w201 = 42 items=["No error", "Argument error", "Memory is full", "Out of zone", "End of file", "File already open", "Generic file I/O error", "File not found", "File permission error", "Disk is full", "Duplicate path", "Too many files open", "System feature not enabled", "Resource file not found", "Cannot add resource", "Resource not found", "Image not found", "Image memory error", "Pen does not exist", "Config type invalid", "Config token not found", "Config parse error", "Config memory error", "Bad external code format", "Bad external code offset", "External code not present", "Null window", "Destroy window error", "Null menu", "Print aborted", "Bad print record", "Print driver error", "Windows error during printing", "Memory error during printing", "Print dialog error", "Generic print error", "Invalid device refnum", "Device not found", "Device parameter error", "Device unit error", "Cannot open device", "Device call aborted", "Generic error", "Cancelled by user", "Object ID too low", "Object ID too high", "Object not in heap", "Unknown heap", "Unknown object (invalid DefProc)", "Unknown object (DefProc not in table)", "Message out of range", "Invalid (null) method", "Unknown message", "Manager call not supported", "Bad address", "Network operation in progress", "Network operation timed out", "Connection is busy", "Network attribute not supported", "Network error", "Address in use", "System out of memory", "Connection aborted", "Connection refused", "Not connected", "Already connected", "Connection closed", "Initialization error (interapplication manager)", "Bad occurrence", "Wait on unbound occurrence handler", "Occurrence queue overflow", "Datalog type conflict", "Unused", "Unrecognized type (interapplication manager)", "Memory corrupt", "Failed to make temporary DLL", "Old CIN version", "Drag socket not found", "Failed to load drop-object", "Failed to register OLE object", "Failed to release OLE object", "Format specifier type mismatch", "Unknown format specifier", "Too few format specifiers", "Too many format specifiers", "Scan failed", "Newer CIN version", "Error converting to variant", "Runtime menu error", "Password tampered", "Variant attribute not found", "Incompatible variant data type", "Event data is not available", "Event Store is not present", "Occurrence is not found", "Event Queue is not created", "Event info is not available", "Refnum passed is NULL", "Error retrieving Class GUID", "Error retrieving CoClass GUID", "Error retrieving TypeLib GUID.", "Bad built application magic bytes.", "Specific driver is different from the specific driver associated with the Logical Name.", "There is no session opened to the class driver.", "Max Error", "MAX - Error with config objects", "MAX - Error loading configuration", "MAX - Group not supported"]
        # "Current State"
        # "Do not delete, rename, or modify this frame.\n(this is used to capture unhandled states and typos)"
        # "Handle mistyped state name (developer tool)"
        n95 = Format Into String(format string="Software Exception: Unhandled State \"%s\"." ("message"), error in=w197, w192) -> (resulting string=w200:string, error out=w199:errorcluster)  [unwired: 1 in]
        n96 = call <vilib>:"Error Cluster From Error Code.vi"("show call chain? (False)"=TRUE, "error in (no error)"=w199, "error message (\"\")"=w200, "error code (0)"=w201) -> ("error out"=w198:errorcluster)  [unwired: 5 in]
        n97 = call <vilib>:"Add State(s) to Queue__jki_lib_state_machine.vi"("State(s) in (\"\")"=w196) -> ("States Out"=w195:string)  [unwired: 14 in]
      }
      frame "Initialize Core Data" {
        # "Do not delete, rename, or modify this frame.\n(this is used to determine panel behavior on exit)"
        # "originally closed?"
        # "exe?"
        # "If panel starts closed or is an EXE, then close it when we exit"
        n98 = property class="VI"() -> ("FP.State"=w205:T5)  [unwired: 2 in, 2 out]
        n99 = property class="App"() -> ("App.Kind"=w211:T6)  [unwired: 2 in, 2 out]
        n100 = control-ref of="Current VI Reference"() -> (w206:refnum<vi>)
        n101 = Equal?(x=w205, y=T5."Closed" ("Front Panel Window:State")) -> (x = y?=w203:bool)
        n102 = Equal?(x=w211, y=T6."Run Time System" ("Application:Kind")) -> (x = y?=w209:bool)
        n103 = Or(x=w203, y=w209) -> (x .or. y?=w207:bool)
        n104 = Bundle By Name(cluster=w208, "Core.Current VI Reference"=w206, "Core.Close Panel on Exit?"=w207) -> (w213:T7)
        n105 = call <vilib>:"Add State(s) to Queue__jki_lib_state_machine.vi"("State(s) in (\"\")"=w215) -> ("States Out"=w214:string)  [unwired: 14 in]
      }
      frame "Error Handler" {
        # "Unhandled Error -- Display it"
        # "Handle any errors here.\nYou can also output any states to clean-up after errors occur"
        # "Clear error"
        n106 = call <vilib>:"General Error Handler.vi"("error in (no error)"=w217) -> ()  [unwired: 10 in, 5 out]
        n107 = call <vilib>:"Add State(s) to Queue__jki_lib_state_machine.vi"("State(s) in Front (\"\")"="/* Post Error States", "State(s) in (\"\")"=w221) -> ("States Out"=w220:string)  [unwired: 13 in]
      }
      frame "Exit" {
        # "Do not put any code in this frame.\n(No errors that occur here will be handled.)"
        n108 = call <vilib>:"Add State(s) to Queue__jki_lib_state_machine.vi"("State(s) in (\"\")"=w226) -> ("States Out"=w225:string)  [unwired: 14 in]
      }
      frame "---------- Data ----------" {
        # "Do not put any code in this frame.\n(It is a separator no-op. You can make a copy of this frame to create a new Data frame)"
        n109 = call <vilib>:"Add State(s) to Queue__jki_lib_state_machine.vi"("State(s) in (\"\")"=w230) -> ("States Out"=w229:string)  [unwired: 14 in]
      }
      frame "Data: Initialize" {
        w243 = T9 {"Current VI Reference"=refnum, "Close Panel on Exit?"=FALSE}  # Core
        w245 = TRUE  # Your Boolean data
        w244 = ""  # String
        # "do not delete - used by framework"
        # "Add new data here."
        # "Data names and types of shift register data are defined by this bundle."
        # "Initialize the shift-register data, here.\n(data names are defined by what you wire into the bundle function)"
        n110 = local read "Queue Table Control"() -> (w240:string[][])
        n111 = local read "Preset Table Control"() -> (w241:string[][])
        n112 = local read "Currently Loaded"() -> (w231:string)
        n113 = property on="Headers" class="Tbl (strict)"() -> ("Column Headers[]"=w242:string[])  [unwired: 2 in, 2 out]
        n114 = call "PresetExecutionDataCluster.vi"() -> ("Preset Manager Cluster"=w239:T10)  [unwired: 1 in]
        n115 = Bundle("Core"=w243, "Your Boolean data"=w245, "String"=w244, "Preset Table Control"=w241, "Column Headers[]"=w242, "Queue Table Control"=w240, "Preset Manager Cluster"=w239, "Currently Loaded"=w231) -> (w238:T7)  [unwired: 1 in]
        n116 = Bundle By Name(cluster=w238, "Preset Manager Cluster.DevStatusQueue"="DevStatusQueue", "Preset Manager Cluster.Experiment Name"="Experiment Name", "Preset Manager Cluster.Software Root"="Software Root", "Preset Manager Cluster.Filtered Devices List"="Filtered Devices List", "Preset Manager Cluster.Virtual Devices List"="Virtual Devices List") -> (w237:T7)
        n117 = call <vilib>:"Add State(s) to Queue__jki_lib_state_machine.vi"("State(s) in (\"\")"=w248) -> ("States Out"=w247:string)  [unwired: 14 in]
      }
      frame "Data: Cleanup" {
        # "Cleanup any data and references, here.\n(this is called automatically, by the Macro: Exit)"
        n118 = Unbundle By Name(w249) -> ("Core.Current VI Reference"=w252:refnum<vi>)
        n119 = Close Reference(reference=w252, error in (no error)=w251) -> (error out=w250:errorcluster)
        n120 = call <vilib>:"Add State(s) to Queue__jki_lib_state_machine.vi"("State(s) in (\"\")"=w254) -> ("States Out"=w253:string)  [unwired: 14 in]
      }
      frame "---------- UI ----------" {
        # "Do not put any code in this frame.\n(It is a separator no-op. You can make a copy of this frame to create a new UI frame)"
        n121 = call <vilib>:"Add State(s) to Queue__jki_lib_state_machine.vi"("State(s) in (\"\")"=w258) -> ("States Out"=w257:string)  [unwired: 14 in]
      }
      frame "UI: Initialize" {
        # "Initialize the User Interface, here.\n(this is called automatically, by the Macro: Init)"
        n122 = call <vilib>:"Add State(s) to Queue__jki_lib_state_machine.vi"("State(s) in (\"\")"=w262) -> ("States Out"=w261:string)  [unwired: 14 in]
      }
      frame "UI: Cursor Set" {
        # "Argument"
        # "Set and Unset Cursor Busy.\n(Usage: \"UI: Cursor Set >> Busy|Idle\")"
        n123 = case shown="\"Idle\", Default" w263 {
          tunnel: w265 -> [w270 w272]
          tunnel: [w269 w271] -> w264
          frame "Idle", Default {
            n124 = call <vilib>:"Unset Busy.vi"("error in (no error)"=w270) -> ("error out"=w269:errorcluster)  [unwired: 10 in]
          }
          frame "Busy" {
            n125 = call <vilib>:"Set Busy.vi"("error in (no error)"=w272) -> ("error out"=w271:errorcluster)  [unwired: 9 in, 1 out]
          }
        }
        n126 = call <vilib>:"Add State(s) to Queue__jki_lib_state_machine.vi"("State(s) in (\"\")"=w268) -> ("States Out"=w267:string)  [unwired: 14 in]
      }
      frame "UI: Front Panel State" {
        # "Argument"
        # "Set Front Panel Open or Closed\n(Usage: \"UI: Front Panel State >> Open|Close\")"
        n127 = Unbundle By Name(w275) -> ("Core.Current VI Reference"=w274:refnum<vi>)
        n128 = case shown="\"Minimize\", \"Minimized\"" w273 {
          tunnel: w277 -> [w285 w300 w311 w324 w337]
          tunnel: [w287 w301 w313 w326 w339] -> w276
          tunnel: w274 -> [w286 w298 w312 w325 w338]
          frame "Open", "Standard", Default {
            w280 = T5."Standard" ("State")
            n129 = property class="VI"(reference=w286, error in=w285) -> (reference out=w283:refnum<vi>, error out=w284:errorcluster, "FP.State"=w282:T5)
            n130 = Not Equal?(x=w282, y=w280) -> (x != y?=w281:bool)
            n131 = case shown="True" w281 {
              tunnel: [w291 w293] -> w287
              tunnel: w284 -> [w290 w293]
              tunnel: w283 -> [w289 _]
              tunnel: w280 -> [w288 _]
              frame True {
                n132 = invoke class="VI" method="FP.Open"(reference=w289, error in=w290, "Activate"=TRUE, "State"=w288) -> (error out=w291:errorcluster)  [unwired: 1 in, 4 out]
              }
              frame False {
              }
            }
          }
          frame "Close", "Closed" {
            n133 = property class="VI"(reference=w298, error in=w300) -> (reference out=w297:refnum<vi>, error out=w299:errorcluster, "FP.State"=w295:T5)
            n134 = Not Equal?(x=w295, y=T5."Closed" ("Front Panel Window:State")) -> (x != y?=w294:bool)
            n135 = case shown="True" w294 {
              tunnel: [w302 w305] -> w301
              tunnel: w299 -> [w302 w304]
              tunnel: w297 -> [_ w303]
              frame False {
              }
              frame True {
                n136 = invoke class="VI" method="FP.Close"(reference=w303, error in=w304) -> (error out=w305:errorcluster)  [unwired: 1 in, 2 out]
              }
            }
          }
          frame "Hidden", "Hide" {
            w306 = T5."Hidden" ("State")
            n137 = property class="VI"(reference=w312, error in=w311) -> (reference out=w309:refnum<vi>, error out=w310:errorcluster, "FP.State"=w308:T5)
            n138 = Not Equal?(x=w308, y=w306) -> (x != y?=w307:bool)
            n139 = case shown="True" w307 {
              tunnel: [w317 w318] -> w313
              tunnel: w310 -> [w316 w318]
              tunnel: w309 -> [w315 _]
              tunnel: w306 -> [w314 _]
              frame True {
                n140 = invoke class="VI" method="FP.Open"(reference=w315, error in=w316, "State"=w314) -> (error out=w317:errorcluster)  [unwired: 2 in, 4 out]
              }
              frame False {
              }
            }
          }
          frame "Minimize", "Minimized" {
            w319 = T5."Minimized" ("State")
            n141 = property class="VI"(reference=w325, error in=w324) -> (reference out=w322:refnum<vi>, error out=w323:errorcluster, "FP.State"=w321:T5)
            n142 = Not Equal?(x=w321, y=w319) -> (x != y?=w320:bool)
            n143 = case shown="True" w320 {
              tunnel: [w330 w331] -> w326
              tunnel: w323 -> [w329 w331]
              tunnel: w322 -> [w328 _]
              tunnel: w319 -> [w327 _]
              frame True {
                n144 = invoke class="VI" method="FP.Open"(reference=w328, error in=w329, "State"=w327) -> (error out=w330:errorcluster)  [unwired: 2 in, 4 out]
              }
              frame False {
              }
            }
          }
          frame "Maximize", "Maximized" {
            w332 = T5."Maximized" ("State")
            n145 = property class="VI"(reference=w338, error in=w337) -> (reference out=w335:refnum<vi>, error out=w336:errorcluster, "FP.State"=w334:T5)
            n146 = Not Equal?(x=w334, y=w332) -> (x != y?=w333:bool)
            n147 = case shown="True" w333 {
              tunnel: [w343 w344] -> w339
              tunnel: w336 -> [w342 w344]
              tunnel: w335 -> [w341 _]
              tunnel: w332 -> [w340 _]
              frame True {
                n148 = invoke class="VI" method="FP.Open"(reference=w341, error in=w342, "State"=w340) -> (error out=w343:errorcluster)  [unwired: 2 in, 4 out]
              }
              frame False {
              }
            }
          }
        }
        n149 = call <vilib>:"Add State(s) to Queue__jki_lib_state_machine.vi"("State(s) in (\"\")"=w279) -> ("States Out"=w278:string)  [unwired: 14 in]
      }
      frame "---------- Macro ----------" {
        # "Do not put any code in this frame.\n(It is a separator no-op. You can make a copy of this frame to create a new Macro frame)"
        n150 = call <vilib>:"Add State(s) to Queue__jki_lib_state_machine.vi"("State(s) in (\"\")"=w348) -> ("States Out"=w347:string)  [unwired: 14 in]
      }
      frame "Macro: Initialize" {
        w349 = string[] [] ("Item Names")
        w354 = 0
        w353 = string[][] [] ("Queue Table")
        w357 = "Data: Initialize\nInitialize Core Data\nUI: Initialize\nUI: Front Panel State >> Open\nInitialize UDP Variables\n Init:PresetMenu\nLoad Preset from DB "  # Data: Initialize Initialize Core Data UI: Initialize UI: Front Panel State >> Open Initialize UDP Variables  Init:PresetMenu Load Preset from DB
        # "Initialization Macro\n(This is called once, when the VI starts)"
        n151 = property on="Queue Size" class="DigNum (strict)"("Value"=w354) -> ()  [unwired: 2 in, 2 out]
        n152 = property on="Queue Element" class="DigNum (strict)"("Value"=w354) -> ()  [unwired: 2 in, 2 out]
        n153 = property on="Preset Table Control" class="Tbl (strict)"("Value"=w353) -> ()  [unwired: 2 in, 2 out]
        n154 = property on="Queue Table" class="Tbl (strict)"("Value"=w353) -> ()  [unwired: 2 in, 2 out]
        n155 = property on="Preset Devices Not in Experiment" class="LstBox (strict)"("Item Names"=w349) -> ()  [unwired: 2 in, 2 out]
        n156 = property on="Preset Devices Not On" class="LstBox (strict)"("Item Names"=w349) -> ()  [unwired: 2 in, 2 out]
        n157 = property on="Preset Menu" class="Ring (strict)"("Strings []"=string[] []) -> ()  [unwired: 2 in, 2 out]
        n158 = property on="Select an ECS file" class="Path"("Value"=path "" ("Select an ECS file")) -> ()  [unwired: 2 in, 2 out]
        n159 = property on="Preset Execution Indicator" class="Bool (strict)"("Blinking"=FALSE, "Caption.Text"="" ("Boolean Text.Text"), "Colors [4]"=cluster{u32, u32}[] [{32639, 0}]) -> ()  [unwired: 2 in, 2 out]
        n160 = call <vilib>:"Add State(s) to Queue__jki_lib_state_machine.vi"("State(s) in Front (\"\")"=w357, "State(s) in (\"\")"=w361) -> ("States Out"=w360:string)  [unwired: 13 in]
      }
      frame "Macro: Exit" {
        # "Exit Macro\n(This is called once, when the VI exits)"
        n161 = Unbundle By Name(w368) -> ("Core.Close Panel on Exit?"=w367:bool)
        n162 = Select(t="UI: Front Panel State >> Close", s=w367, f="") -> (s? t:f=w364:string)
        n163 = call <vilib>:"Add State(s) to Queue__jki_lib_state_machine.vi"("State(s) in (\"\")"=w364, "State(s) at Back (\"\")"="Data: Cleanup\nExit") -> ("States Out"=w362:string)  [unwired: 13 in]
        n164 = call <vilib>:"Add State(s) to Queue__jki_lib_state_machine.vi"("State(s) in Front (\"\")"=w362, "State(s) in (\"\")"=w371) -> ("States Out"=w370:string)  [unwired: 13 in]
      }
      frame "Initialize UDP Variables" {
        # "Do not put any code in this frame.\n(It is a separator no-op. You can make a copy of this frame to create a new Macro frame)"
        n165 = Unbundle By Name(w380) -> ("Preset Manager Cluster.Experiment Name"=w378:string)
        n166 = call "UPD Variable Init.vi"("Expt Name"=w378) -> ("Mcast Address"=w374:string, "UDP timeout ms"=w375:i32, "MC Multicast"=w376:refnum<k16>, "My IP"=w377:string, "Mcast remote"=w373:u16, "> Name, devtype, ip, dev comm port, class, location for all devices>"=w372:string[][])  [unwired: 5 in]
        n167 = Bundle By Name(cluster=w380, "Preset Manager Cluster.My IP"=w377, "Preset Manager Cluster.MC Multicast"=w376, "Preset Manager Cluster.UDP timeout ms"=w375, "Preset Manager Cluster.Mcast address"=w374, "Preset Manager Cluster.MCast Remote"=w373, "Preset Manager Cluster.All Devices Core Info"=w372) -> (w379:T7)
        n168 = call <vilib>:"Add State(s) to Queue__jki_lib_state_machine.vi"("State(s) in (\"\")"=w383) -> ("States Out"=w382:string)  [unwired: 14 in]
      }
      frame "Init:PresetMenu" {
        # "Template Separator\n(You can make a copy of, or modify, this frame)"
        n169 = call "preset SQL Queries.vi"("Preset Query"=Preset_Query_Enum."GetAllPresetNames") -> ("1st column 1st data"=w386:string[])  [unwired: 8 in, 2 out]
        n170 = Sort 1D Array(array=w386) -> (sorted array=w385:string[])
        n171 = control-ref of="Preset Menu"() -> (w387:refnum<vi>)
        n172 = Insert Into Array(array=w385, index=0, new element="None" ("new element/subarray")) -> (w384:string[])
        n173 = property on="Property Node" class="Ring (strict)"(reference=w387, "Strings []"=w384, "Value"=0 ("index")) -> ()  [unwired: 1 in, 2 out]
        n174 = call <vilib>:"Add State(s) to Queue__jki_lib_state_machine.vi"("State(s) in Front (\"\")"="Implement Value Change" ("State(s) in Front (\"\")"), "State(s) in (\"\")"=w396) -> ("States Out"=w395:string)  [unwired: 13 in]
      }
      frame "---------- Menu Control ----------" {
        # "Template Separator\n(You can make a copy of, or modify, this frame)"
        n175 = call <vilib>:"Add State(s) to Queue__jki_lib_state_machine.vi"("State(s) in (\"\")"=w400) -> ("States Out"=w399:string)  [unwired: 14 in]
      }
      frame "Compare Table" {
        # "Template Separator\n(You can make a copy of, or modify, this frame)"
        n176 = property on="PRESET FROM DB" class="Tbl (strict)"() -> ("Value"=w411:string[][])  [unwired: 2 in, 2 out]
        n177 = property on="ECS File" class="Tbl (strict)"() -> ("Value"=w410:string[][])  [unwired: 2 in, 2 out]
        n178 = Unbundle By Name(w405) -> ("Preset Manager Cluster.PresetName"=w402:string, "Currently Loaded"=w403:string)
        n179 = call "Left Join.vi"("Array 2"=w410, "Array 1"=w411) -> ("Left Joined Array"=w409:string[][])  [unwired: 9 in]
        n180 = Concatenate Strings(w402, " joined with " ("string"), w403) -> (w404:string)
        n181 = Bundle By Name(cluster=w405, "Preset Table Control"=w409, "Column Headers[]"=string[] ["Device Name", "Device Variable", "Preset Value", "ECS Value"] ("Column Headers")) -> (w408:T7)
        n182 = local write "Currently Loaded"(w404) -> ()
        n183 = call <vilib>:"Add State(s) to Queue__jki_lib_state_machine.vi"("State(s) in Front (\"\")"="Table Update" ("State(s) in Front (\"\")"), "State(s) in (\"\")"=w414) -> ("States Out"=w413:string)  [unwired: 13 in]
      }
      frame "Choose Values" {
        # "Template Separator\n(You can make a copy of, or modify, this frame)"
        n184 = property on="Preset Table Control" class="Tbl (strict)"() -> ("Value"=w418:string[][])  [unwired: 2 in, 2 out]
        n185 = call "Value_Selection_in_Table_GUI.vi"("Column Headers"=string[] ["Device Name", "Device Variable", "Preset Value", "ECS Value"], "SELECTION TABLE - Click on values to keep"=w418) -> ("Coordinate Array"=→"Coordinate Array":i32[][])  [unwired: 9 in]
        n186 = call <vilib>:"Add State(s) to Queue__jki_lib_state_machine.vi"("State(s) in Front (\"\")"="Implement Value Change" ("State(s) in Front (\"\")"), "State(s) in (\"\")"=w422) -> ("States Out"=w421:string)  [unwired: 13 in]
      }
      frame "Preset Builder" {
        # "Template Separator\n(You can make a copy of, or modify, this frame)"
        n187 = Unbundle By Name(w428) -> ("Preset Table Control"=w426:string[][], "Column Headers[]"=w425:string[])
        n188 = call "Preset Builder.vi"("Column Header"=w425, "Input Table"=w426) -> ("Exit Indicator"=w423:bool, "Output Table"=w424:string[][])  [unwired: 7 in]
        n189 = Bundle By Name(cluster=w428, "Preset Table Control"=w424) -> (w427:T7)
        n190 = case shown="True" w423 {
          frame False {
          }
          frame True {
            n191 = local write "Currently Loaded"("Output from preset builder" ("Currently Loaded")) -> ()
          }
        }
        n192 = call <vilib>:"Add State(s) to Queue__jki_lib_state_machine.vi"("State(s) in Front (\"\")"="Table Update" ("State(s) in Front (\"\")"), "State(s) in (\"\")"=w432) -> ("States Out"=w431:string)  [unwired: 13 in]
      }
      frame "Implement Value Change" {
        # "Template Separator\n(You can make a copy of, or modify, this frame)"
        n193 = Unbundle By Name(w440) -> ("Preset Table Control"=w438:string[][])
        n194 = property on="Coordinate Array" class="Arr (strict)"() -> ("Value"=w437:i32[][])  [unwired: 2 in, 2 out]
        n195 = call "Value_Update_to_Preset.vi"("Coordinate Array with Changes"=w437, "Input Table"=w438) -> ("Column Headers"=w435:string[], "Output Table with Changes"=w436:string[][])  [unwired: 8 in]
        n196 = Bundle By Name(cluster=w440, "Preset Table Control"=w436, "Column Headers[]"=w435) -> (w439:T7)
        n197 = local write "Currently Loaded"("Table with Chosen Values" ("Currently Loaded")) -> ()
        n198 = call <vilib>:"Add State(s) to Queue__jki_lib_state_machine.vi"("State(s) in Front (\"\")"="Table Update" ("State(s) in Front (\"\")"), "State(s) in (\"\")"=w444) -> ("States Out"=w443:string)  [unwired: 13 in]
      }
      frame "Load Preset from DB" {
        # "Template Separator\n(You can make a copy of, or modify, this frame)"
        n199 = property on="Preset Menu" class="Ring (strict)"() -> ("RingText.Text"=w445:string)  [unwired: 2 in, 2 out]
        n200 = call "Preset_to_Array.vi"("Preset Name"=w445) -> ("Column Headers"=w447:string[], "Preset Table"=w446:string[][])  [unwired: 9 in]
        "PRESET FROM DB" <- w446
        n201 = Bundle By Name(cluster=w450, "Preset Table Control"=w446, "Column Headers[]"=w447, "Preset Manager Cluster.PresetName"=w445) -> (w449:T7)
        n202 = local write "Currently Loaded"(w445) -> ()
        n203 = call <vilib>:"Add State(s) to Queue__jki_lib_state_machine.vi"("State(s) in Front (\"\")"="Table Update\nExpt Device Check>>Preset Only" ("State(s) in Front (\"\")"), "State(s) in (\"\")"=w453) -> ("States Out"=w452:string)  [unwired: 13 in]
      }
      frame "Load Configuration File" {
        # "Template Separator\n(You can make a copy of, or modify, this frame)"
        n204 = call <vilib>:"Add State(s) to Queue__jki_lib_state_machine.vi"("State(s) in Front (\"\")"="Table Update" ("State(s) in Front (\"\")"), "State(s) in (\"\")"=w467) -> ("States Out"=w466:string)  [unwired: 13 in]
        n205 = Path To String(path="Select an ECS file") -> (string=w459:string)
        n206 = xnode "Match Regular Expression"("input string"=w459, "regular expression"="([^\\\\/]+\\.txt)$") -> ("whole match"=w457:string)  [unwired: 4 in, 4 out]
        n207 = Match Pattern(string=w457, regular expression=".txt") -> (before substring=w454:string)  [unwired: 1 in, 3 out]
        n208 = call "Configuration_to_Array.vi"("file (use dialog)"="Select an ECS file") -> ("Table Control"=w462:string[][])  [unwired: 10 in]
        "ECS File" <- w462
        n209 = Bundle By Name(cluster=w464, "Preset Table Control"=w462, "Column Headers[]"=string[] ["Device Name", "Device Variable", "ECS Values"] ("Column Headers"), "Currently Loaded"=w454) -> (w463:T7)
        n210 = local write "Currently Loaded"(w454) -> ()
      }
      frame "Save Preset" {
        # "Template Separator\n(You can make a copy of, or modify, this frame)"
        n211 = Unbundle By Name(w582) -> ("Preset Manager Cluster.PresetName"=w583:string)
        n212 = Concatenate Strings("Overwrite " ("Right Button Text (\"Cancel\")"), w583) -> (w584:string)
        n213 = call <vilib>:"Three Button Dialog.vi"("Right Button Text (\"Cancel\")"="Cancel" ("Right Button Text (\"Cancel\")"), "Center Button Text (\"No\")"=w584, "Left Button Text (\"Yes\")"="Save as New Preset" ("Left Button Text (\"Yes\")"), "message"="Save the current preset as - ") -> ("Which Button?"=w587:T11)  [unwired: 7 in]
        n214 = case shown="\"Right Button\", Default" w587 {
          tunnel: ["Save as New Preset" ("State(s) in Front (\"\")") "Overwrite Existing Preset" ("Right Button Text (\"Cancel\")") _] -> w586
          frame "Left Button" {
          }
          frame "Center Button" {
          }
          frame "Right Button", Default {
          }
        }
        n215 = call <vilib>:"Add State(s) to Queue__jki_lib_state_machine.vi"("State(s) in Front (\"\")"=w586, "State(s) in (\"\")"=w593) -> ("States Out"=w592:string)  [unwired: 13 in]
      }
      frame "Save as New Preset" {
        # "Template Separator\n(You can make a copy of, or modify, this frame)"
        n216 = call "Preset Name"() -> ("Name"=w597:string, "OK"=w606:bool)  [unwired: 17 in, 1 out]
        n217 = property on="Preset Menu" class="Ring (strict)"() -> ("Strings []"=w603:string[])  [unwired: 2 in, 2 out]
        n218 = Search 1D Array(1D array=w603, element=w597) -> (index of element=w602:i32)  [unwired: 1 in]
        n219 = call <vilib>:"Trim Whitespace.vi"("string"=w597) -> ("trimmed string"=w605:string)  [unwired: 1 in]
        n220 = Equal?(x=w605, y="") -> (x = y?=w600:bool)
        n221 = Not Equal?(x=w602, y=-1) -> (x != y?=w599:bool)
        n222 = Or(x=w600, y=w599) -> (x .or. y?=w598:bool)
        n223 = case shown="True" w606 {
          tunnel: w598 -> [_ w612]
          tunnel: w597 -> [_ w611]
          frame False {
          }
          frame True {
            n224 = case shown="False" w612 {
              tunnel: w611 -> [w613 _]
              frame False {
                n225 = stacked-sequence {
                  tunnel: w613 -> [w615]
                  frame #0 {
                    n226 = local read "Preset Table Control"() -> (w614:string[][])
                    n227 = for {
                      tunnel: w615 -> [w620]
                      tunnel: w614 -> [w616] mode=indexing
                      n228 = Insert Into Array(array=w616, index=0, new element=w620) -> (w618:string[])
                      n229 = call "SQL Insert null.vi"("Values"=w618, "Column Names"=string[] ["presetName", "presetDevice", "presetVariable", "presetValue"], "Table"="Presets") -> ("Query String"=w617:string)  [unwired: 8 in]
                      n230 = disable-structure shown="Enabled" {
                        disable-tunnel: w617 -> [w623 _]
                        frame Enabled {
                          n231 = call "SQL Server Info.vi"() -> ("SQL Server Info"=w624:T13)
                          n232 = call "SQL Query.vi"("SQL Server Info"=w624, "Query"=w623) -> ()  [unwired: 8 in, 2 out]
                        }
                        frame Disabled {
                        }
                      }
                    }
                  }
                }
              }
              frame True {
                n233 = One Button Dialog(message="Name field was blank or the Preset Name already exists") -> ()  [unwired: 1 in, 1 out]
              }
            }
          }
        }
        n234 = call <vilib>:"Add State(s) to Queue__jki_lib_state_machine.vi"("State(s) in Front (\"\")"="Load Preset from DB>>Table Update" ("State(s) in Front (\"\")"), "State(s) in (\"\")"=w610) -> ("States Out"=w609:string)  [unwired: 13 in]
      }
      frame "Overwrite Existing Preset" {
        # "Template Separator\n(You can make a copy of, or modify, this frame)"
        n235 = property on="Preset Menu" class="Ring (strict)"() -> ("RingText.Text"=w627:string)  [unwired: 2 in, 2 out]
        n236 = Concatenate Strings("Are you sure you want to overwrite " ("string"), w627, " with the current table ?" ("string")) -> (w630:string)
        n237 = Two Button Dialog(message=w630, 2:"Yes" ("T button name (\"OK\")")) -> (T button?=w628:bool)  [unwired: 1 in]
        n238 = case shown="True" w628 {
          tunnel: w627 -> [_ w637]
          frame False {
          }
          frame True {
            n239 = stacked-sequence {
              seq-local: [w638 _] -> [_ w648]
              tunnel: w637 -> [w639 w647]
              tunnel: [_ w648] -> _
              frame #0 {
                n240 = disable-structure shown="Enabled" {
                  disable-tunnel: w639 -> [w643 _]
                  disable-tunnel: [w640 _] -> w638
                  frame Enabled {
                    n241 = Concatenate Strings("DELETE FROM Presets WHERE presetName='", w643, "'" ("string")) -> (w641:string)
                    n242 = call "SQL Server Info.vi"() -> ("SQL Server Info"=w645:T13)
                    n243 = call "SQL Query.vi"("SQL Server Info"=w645, "Query"=w641) -> ("error out"=w640:errorcluster)  [unwired: 8 in, 1 out]
                  }
                  frame Disabled {
                  }
                }
              }
              frame #1 {
                n244 = local read "Preset Table Control"() -> (w646:string[][])
                n245 = for {
                  tunnel: w648 -> [w656]
                  tunnel: w647 -> [w653]
                  tunnel: w646 -> [w649] mode=indexing
                  n246 = Insert Into Array(array=w649, index=0, new element=w653) -> (w651:string[])
                  n247 = call "SQL Insert null.vi"("Values"=w651, "Column Names"=string[] ["presetName", "presetDevice", "presetVariable", "presetValue"], "Table"="Presets") -> ("Query String"=w650:string)  [unwired: 8 in]
                  n248 = disable-structure shown="Enabled" {
                    disable-tunnel: w656 -> [w658 _]
                    disable-tunnel: w650 -> [w657 _]
                    frame Enabled {
                      n249 = call "SQL Server Info.vi"() -> ("SQL Server Info"=w659:T13)
                      n250 = call "SQL Query.vi"("error in (no error)"=w658, "SQL Server Info"=w659, "Query"=w657) -> ()  [unwired: 7 in, 2 out]
                    }
                    frame Disabled {
                    }
                  }
                }
              }
            }
          }
        }
        n251 = call <vilib>:"Add State(s) to Queue__jki_lib_state_machine.vi"("State(s) in Front (\"\")"="Load Preset from DB>>Table Update" ("State(s) in Front (\"\")"), "State(s) in (\"\")"=w636) -> ("States Out"=w635:string)  [unwired: 13 in]
      }
      frame "Delete Preset" {
        # "Template Separator\n(You can make a copy of, or modify, this frame)"
        n252 = property on="Preset Menu" class="Ring (strict)"() -> ("RingText.Text"=w660:string)  [unwired: 2 in, 2 out]
        n253 = Concatenate Strings("Are you sure you want to delete " ("string"), w660, ". NOTE - THIS ACTION IS NOT REVERSIBLE" ("string")) -> (w663:string)
        n254 = Two Button Dialog(message=w663, 2:"Yes" ("T button name (\"OK\")")) -> (T button?=w661:bool)  [unwired: 1 in]
        n255 = case shown="True" w661 {
          tunnel: w660 -> [_ w671]
          frame False {
          }
          frame True {
            n256 = stacked-sequence {
              tunnel: w671 -> [w672 _]
              frame #0 {
                n257 = disable-structure shown="Enabled" {
                  disable-tunnel: w672 -> [w677 _]
                  frame Enabled {
                    n258 = Concatenate Strings("DELETE FROM Presets WHERE presetName='", w677, "'" ("string")) -> (w673:string)
                    n259 = call "SQL Server Info.vi"() -> ("SQL Server Info"=w676:T13)
                    n260 = call "SQL Query.vi"("SQL Server Info"=w676, "Query"=w673) -> ()  [unwired: 8 in, 2 out]
                  }
                  frame Disabled {
                  }
                }
              }
              frame #1 {
              }
            }
          }
        }
        n261 = call <vilib>:"Add State(s) to Queue__jki_lib_state_machine.vi"("State(s) in Front (\"\")"="Load Preset from DB>>Table Update" ("State(s) in Front (\"\")"), "State(s) in (\"\")"=w670) -> ("States Out"=w669:string)  [unwired: 13 in]
      }
      frame "Execute Preset" {
        # "Template Separator\n(You can make a copy of, or modify, this frame)"
        n262 = case shown="False" "Dont jump \nto diagnostics" {
          frame False {
            n263 = property on="Tab Control" class="TabCtl (strict)"("Value"=T1."Diagnostics" ("Tab Control")) -> ()  [unwired: 2 in, 2 out]
          }
          frame True {
          }
        }
        n264 = control-ref of="Preset Execution Indicator"() -> (w683:refnum<vi>)
        n265 = local write "Abort Execution"(T2 FALSE ("Abort Execution")) -> ()
        n266 = property on="Property Node" class="Bool (strict)"(reference=w683, "Blinking"=TRUE, "Caption.Text"="Executing Preset" ("Boolean Text.Text")) -> ()  [unwired: 1 in, 2 out]
        n267 = call <vilib>:"Add State(s) to Queue__jki_lib_state_machine.vi"("State(s) in Front (\"\")"="Send Preset Command" ("State(s) in Front (\"\")"), "State(s) in (\"\")"=w687) -> ("States Out"=w686:string)  [unwired: 13 in]
      }
      frame "-------Table Update--------" {
        # "Template Separator\n(You can make a copy of, or modify, this frame)"
        n268 = call <vilib>:"Add State(s) to Queue__jki_lib_state_machine.vi"("State(s) in (\"\")"=w692) -> ("States Out"=w691:string)  [unwired: 14 in]
      }
      frame "Table Update" {
        # "Template Separator\n(You can make a copy of, or modify, this frame)"
        n269 = Unbundle By Name(w695) -> ("Preset Table Control"=w694:string[][], "Column Headers[]"=w693:string[])
        n270 = property on="Preset Table Control" class="Tbl (strict)"("Value"=w694, "Column Headers[]"=w693) -> ()  [unwired: 2 in, 2 out]
        n271 = call <vilib>:"Add State(s) to Queue__jki_lib_state_machine.vi"("State(s) in (\"\")"=w698) -> ("States Out"=w697:string)  [unwired: 14 in]
      }
      frame "--------Queue Presets------------" {
        # "Template Separator\n(You can make a copy of, or modify, this frame)"
        n272 = call <vilib>:"Add State(s) to Queue__jki_lib_state_machine.vi"("State(s) in (\"\")"=w702) -> ("States Out"=w701:string)  [unwired: 14 in]
      }
      frame "Load Preset Queue" {
        # "Template Separator\n(You can make a copy of, or modify, this frame)"
        n273 = call-poly <vilib>:"Read Delimited Spreadsheet.vi"("error in (no error)"=w706) -> ("all rows"=w704:string[][], "error out"=w705:errorcluster)  [unwired: 9 in, 4 out]
        n274 = local write "Queue Table"(w704) -> ()
        n275 = call <vilib>:"Add State(s) to Queue__jki_lib_state_machine.vi"("State(s) in (\"\")"=w708) -> ("States Out"=w707:string)  [unwired: 14 in]
      }
      frame "Save Preset Queue" {
        # "Template Separator\n(You can make a copy of, or modify, this frame)"
        n276 = local read "Queue Table"() -> (w709:string[][])
        n277 = call-poly <vilib>:"Write Delimited Spreadsheet.vi"("2D data"=w709, "error in (no error)"=w711) -> ("error out"=w710:errorcluster)  [unwired: 12 in, 1 out]
        n278 = call <vilib>:"Add State(s) to Queue__jki_lib_state_machine.vi"("State(s) in (\"\")"=w714) -> ("States Out"=w713:string)  [unwired: 14 in]
      }
      frame "Init: Queue Preset" {
        # "Template Separator\n(You can make a copy of, or modify, this frame)"
        n279 = property on="Tab Control" class="TabCtl (strict)"() -> ("Value"=w715:T1)  [unwired: 2 in, 2 out]
        n280 = Equal?(x=w715, y=1) -> (x = y?=w718:bool)
        n281 = case shown="True" w718 {
          frame False {
          }
          frame True {
            n282 = call "preset SQL Queries.vi"("Preset Query"=Preset_Query_Enum."GetAllPresetNames") -> ("data"=w726:string[][])  [unwired: 8 in, 2 out]
            n283 = Array Subset(array=w726, index (row)=1 ("index")) -> (w725:string[][])  [unwired: 3 in]
            n284 = call "Sort 2D Array.vim"("index"=0, "dimension to index (column)"=enum16{"column", "row"}."column", "2D array"=w725) -> ("sorted 2D array"=w724:string[][])  [unwired: 7 in, 1 out]
            n285 = property on="Queue Table Control" class="Tbl (strict)"("Value"=w724) -> ()  [unwired: 2 in, 2 out]
          }
        }
        n286 = call <vilib>:"Add State(s) to Queue__jki_lib_state_machine.vi"("State(s) in (\"\")"=w721) -> ("States Out"=w720:string)  [unwired: 14 in]
      }
      frame "Reset Queue" {
        # "Template Separator\n(You can make a copy of, or modify, this frame)"
        n287 = property on="Queue Table" class="Tbl (strict)"("Value"=string[][] [] ("Queue Table")) -> ()  [unwired: 2 in, 2 out]
        n288 = call <vilib>:"Add State(s) to Queue__jki_lib_state_machine.vi"("State(s) in (\"\")"=w733) -> ("States Out"=w732:string)  [unwired: 14 in]
      }
      frame "Execute Queue" {
        # "Template Separator\n(You can make a copy of, or modify, this frame)"
        n289 = flat-sequence {
          frame #0 {
            w740 = TRUE
            n290 = property on="Queue Size" class="DigNum (strict)"("Visible"=w740) -> ()  [unwired: 2 in, 2 out]
            n291 = property on="Current Preset Queue Element" class="Str"("Visible"=w740) -> ()  [unwired: 2 in, 2 out]
            n292 = property on="Queue Progress Bar" class="Slide (strict)"("Visible"=w740) -> ()  [unwired: 2 in, 2 out]
          }
          frame #1 {
            n293 = property on="Queue Table" class="Tbl (strict)"() -> ("Value"=w748:string[][])  [unwired: 2 in, 2 out]
            n294 = property on="Queue Progress Bar" class="Slide (strict)"("Value"=u8 0 ("Queue Progress Bar"), "Maximum"=1.0 ("Data Entry Limits:Maximum")) -> ()  [unwired: 2 in, 2 out]
            n295 = property on="Using Queue" class="Bool (strict)"("Value"=TRUE ("Value (Signaling)")) -> ()  [unwired: 2 in, 2 out]
            n296 = Index Array(array=w748, index (col)=0 ("disabled index (col)")) -> (element=w746:string[])  [unwired: 1 in]
            n297 = Array Size(array=w746) -> (size(s)=→"Queue Size":i32)
            "Queue Element" <- 1 ("Element")
          }
          frame #2 {
          }
        }
        n298 = local write "Abort Execution"(T2 FALSE ("Abort Execution")) -> ()
        n299 = call <vilib>:"Add State(s) to Queue__jki_lib_state_machine.vi"("State(s) in Front (\"\")"="Preset Queue Loading" ("State(s) in Front (\"\")"), "State(s) in (\"\")"=w739) -> ("States Out"=w738:string)  [unwired: 13 in]
      }
      frame "Preset Queue Loading" {
        # "Template Separator\n(You can make a copy of, or modify, this frame)"
        n300 = flat-sequence {
          tunnel: w750 -> [w758]
          tunnel: [w759] -> w751
          tunnel: [w757] -> w749
          frame #0 {
            n301 = property on="Queue Element" class="DigNum (strict)"() -> ("Value"=w756:i32)  [unwired: 2 in, 2 out]
            n302 = property on="Queue Size" class="DigNum (strict)"() -> ("Value"=w755:i32)  [unwired: 2 in, 2 out]
            n303 = Less?(x=w755, y=w756) -> (x < y?=w760:bool)
            n304 = case shown="False" w760 {
              tunnel: [w766 ""] -> w759
              tunnel: w758 -> [w765 w776]
              tunnel: [w764 w776] -> w757
              tunnel: w756 -> [w763 _]
              tunnel: w755 -> [w762 _]
              frame False {
                n305 = Divide(x=w763, y=w762) -> (x/y=w761:dbl)
                n306 = flat-sequence {
                  tunnel: w765 -> [w769]
                  tunnel: [w768] -> w764
                  tunnel: ["Execute Preset"] -> w766
                  frame #0 {
                    n307 = property on="Queue Element" class="DigNum (strict)"() -> ("Value"=w771:i32)  [unwired: 2 in, 2 out]
                    n308 = local read "Queue Table"() -> (w773:string[][])
                    n309 = Decrement(x=w771) -> (x-1=w770:i32)
                    n310 = Index Array(array=w773, index (row)=w770, index (col)=0 ("disabled index (col)")) -> (element=w767:string)
                    "Current Preset Queue Element" <- w767
                    n311 = Bundle By Name(cluster=w769, "Preset Manager Cluster.PresetName"=w767) -> (w768:T7)
                  }
                  frame #1 {
                  }
                }
                n312 = property on="Queue Progress Bar" class="Slide (strict)"("Value"=w761) -> ()  [unwired: 2 in, 2 out]
              }
              frame True {
                n313 = property on="Using Queue" class="Bool (strict)"("Val(Sgnl)"=FALSE ("Value (Signaling)")) -> ()  [unwired: 2 in, 2 out]
              }
            }
          }
        }
        n314 = call <vilib>:"Add State(s) to Queue__jki_lib_state_machine.vi"("State(s) in Front (\"\")"=w751, "State(s) in (\"\")"=w754) -> ("States Out"=w753:string)  [unwired: 13 in]
      }
      frame "-------Preset Execution----------" {
        # "Template Separator\n(You can make a copy of, or modify, this frame)"
        n315 = call <vilib>:"Add State(s) to Queue__jki_lib_state_machine.vi"("State(s) in (\"\")"=w781) -> ("States Out"=w780:string)  [unwired: 14 in]
      }
      frame "General wait" {
        # "Template Separator\n(You can make a copy of, or modify, this frame)"
        n316 = call "get arguments of jki state.vi"("jki arguments"=w782) -> ("Arg 1"=w784:string)  [unwired: 1 in, 2 out]
        n317 = Decimal String To Number(string=w784) -> (number=w783:i32)  [unwired: 2 in, 1 out]
        n318 = Wait (ms)(milliseconds to wait=w783) -> ()  [unwired: 1 out]
        n319 = call <vilib>:"Add State(s) to Queue__jki_lib_state_machine.vi"("State(s) in (\"\")"=w788) -> ("States Out"=w787:string)  [unwired: 14 in]
      }
      frame "Check Abort" {
        # "Template Separator\n(You can make a copy of, or modify, this frame)"
        n320 = case shown="True" "Abort Execution" {
          tunnel: ["Poll Devices" ""] -> w790
          frame False {
          }
          frame True {
            n321 = property on="Preset Execution Indicator" class="Bool (strict)"("Blinking"=FALSE, "Caption.Text"=" Preset Aborted" ("Boolean Text.Text"), "Value"=FALSE ("Blinking"), "Colors [4]"=cluster{u32, u32}[] [{16711680, 0}]) -> ()  [unwired: 2 in, 2 out]
            n322 = property on="Tab Control" class="TabCtl (strict)"("Value"=T1."Diagnostics" ("Tab Control")) -> ()  [unwired: 2 in, 2 out]
          }
        }
        n323 = call <vilib>:"Add State(s) to Queue__jki_lib_state_machine.vi"("State(s) in Front (\"\")"=w790, "State(s) in (\"\")"=w794) -> ("States Out"=w793:string)  [unwired: 13 in]
      }
      frame "Poll Devices" {
        # "rem virt devs"
        # "Template Separator\n(You can make a copy of, or modify, this frame)"
        n324 = Unbundle By Name(w821) -> ("Preset Manager Cluster"=w820:T10)
        n325 = Unbundle By Name(w820) -> ("PresetName"=w807:string, "Current Preset Devices"=w816:string[], "All Devices Core Info"=w819:string[][], "Filtered Devices List"=w818:string[], "Virtual Devices List"=w817:string[], "DevStatusQueue"=w811:refnum<queue>)
        n326 = call "search string array for elements in 2nd string array.vi"("search for"=w817, "search in"=w818) -> ("Indices of Elements"=w822:i32[])  [unwired: 9 in]
        n327 = call-poly <userlib>:"Delete Elements from Array__ogtk.vi"("indices"=w822, "array"=w818) -> ("array w/ subset deleted"=w813:string[])  [unwired: 8 in, 1 out]
        n328 = call "get info from core device data.vi"("devices to get data from"=w813, "All Devices Core Info"=w819) -> ("IP Addresses"=w814:string[])  [unwired: 2 in, 3 out]
        n329 = Empty Array?(array=w814) -> (empty?=w815:bool)
        n330 = Preview Queue Element(queue=w811, timeout in ms (-1)=200) -> (element=w810:string[][], error out=→"error out":errorcluster)  [unwired: 1 in, 2 out]
        n331 = Wait (ms)(milliseconds to wait=u32 500) -> ()  [unwired: 1 out]
        n332 = flat-sequence {
          tunnel: w816 -> [w832]
          tunnel: w815 -> [w831]
          tunnel: w814 -> [w830]
          tunnel: w813 -> [w829]
          tunnel: w810 -> [w828]
          tunnel: w807 -> [w826]
          tunnel: [w827] -> w805
          tunnel: [w826] -> w803
          tunnel: [w858] -> w808
          tunnel: w805 -> [w858]
          tunnel: [w852] -> w804
          tunnel: w803 -> [w851]
          frame #0 {
            n333 = case shown="False" w831 {
              tunnel: w826 -> [w844 _]
              tunnel: w832 -> [w843 _]
              tunnel: w830 -> [w842 _]
              tunnel: w829 -> [w841 _]
              tunnel: w828 -> [w839 _]
              tunnel: [w838 FALSE ("Active Preset Achieved")] -> w827
              frame False {
                # "Determine which devices are ON/OFF"
                n334 = call "get device status from tcp data array.vi"("TCP Device status data"=w839, "Current Preset Devices"=w843, "IP Addresses in"=w842, "Filtered Device List"=w841, "Requested Preset"=w844) -> ("Device Errors"=→"Device Errors":string[][], "Active boolean array"=→"Active Device array":bool[], "preset diagnostics"=w837:T14, "Active IP Addresses"=→"Active Dev/IP":string[], "Devices Not alive"=→"Devices not started":string[])  [unwired: 3 in, 3 out]
                n335 = Unbundle By Name(w837) -> ("Active Preset Achieved"=w838:bool)
                n336 = Unbundle By Name(w837) -> ("Active Preset Achieved"=→"Active Preset Achieved":bool, "Devices with Active Preset Not Set"=→"Devices with Active \nPreset Not Set":string[], "Dev Presets"=→"Dev Presets":string[], "All Preset Devices ON?"=→"All Preset Devices ON?":bool[])
                n337 = Select(t=w844, s=w838, f="Undefined") -> (s? t:f=→"Active Preset":string)
              }
              frame True {
              }
            }
          }
          frame #1 {
            n338 = property on="Active Preset" class="Str"() -> ("Value"=w854:string)  [unwired: 2 in, 2 out]
            n339 = property on="Poll Count" class="DigNum (strict)"() -> ("Value"=w856:i32)  [unwired: 2 in, 2 out]
            n340 = Not Equal?(x=w851, y=w854) -> (x != y?=w855:bool)
            n341 = Less?(x=w856, y=120) -> (x < y?=w857:bool)
            n342 = And(x=w855, y=w857) -> (x .and. y?=w852:bool)
          }
        }
        n343 = case shown="False" w804 {
          tunnel: w808 -> [w860 _]
          tunnel: [w859 "Check Abort"] -> w806
          frame False {
            n344 = case shown="True" w860 {
              tunnel: ["" w866] -> w859
              frame False {
                n345 = property on="Preset Execution Indicator" class="Bool (strict)"("Blinking"=FALSE, "Caption.Text"=" Preset Failed" ("Boolean Text.Text"), "Value"=FALSE ("Blinking"), "Colors [4]"=cluster{u32, u32}[] [{16711680, 0}]) -> ()  [unwired: 2 in, 2 out]
              }
              frame True {
                n346 = disable-structure shown="Enabled" {
                  frame Disabled {
                    n347 = property on="Preset Execution Indicator" class="Bool (strict)"("Blinking"=FALSE, "Caption.Text"=" Preset Executed" ("Boolean Text.Text"), "Value"=TRUE ("Blinking"), "Colors [4]"=cluster{u32, u32}[] [{318464, 0}]) -> ()  [unwired: 2 in, 2 out]
                  }
                  frame Enabled {
                    n348 = property on="Preset Execution Indicator" class="Bool (strict)"("Blinking"=FALSE, "Caption.Text"="Preset Executed" ("Boolean Text.Text"), "Value"=FALSE ("Blinking"), "Colors [4]"=cluster{u32, u32}[] [{499456, 0}]) -> ()  [unwired: 2 in, 2 out]
                  }
                }
                n349 = property on="Using Queue" class="Bool (strict)"() -> ("Value"=w867:bool)  [unwired: 2 in, 2 out]
                n350 = case shown="False" w867 {
                  tunnel: ["" "Preset Queue Loading"] -> w866
                  frame False {
                  }
                  frame True {
                    n351 = property on="Queue Element" class="DigNum (strict)"() -> ("Value"=w879:i32)  [unwired: 2 in, 2 out]
                    n352 = Increment(x=w879) -> (x+1=w878:i32)
                    n353 = property on="Queue Element" class="DigNum (strict)"("Value"=w878) -> ()  [unwired: 2 in, 2 out]
                  }
                }
              }
            }
          }
          frame True {
            n354 = property on="Poll Count" class="DigNum (strict)"() -> ("Value"=w882:i32)  [unwired: 2 in, 2 out]
            n355 = Increment(x=w882) -> (x+1=w881:i32)
            n356 = property on="Poll Count" class="DigNum (strict)"("Value"=w881) -> ()  [unwired: 2 in, 2 out]
          }
        }
        n357 = call <vilib>:"Add State(s) to Queue__jki_lib_state_machine.vi"("State(s) in Front (\"\")"=w806, "State(s) in (\"\")"=w825) -> ("States Out"=w824:string)  [unwired: 13 in]
      }
      frame "Send Preset Command" {
        # "This State builds the Multicast Preset Command to all Devices"
        # "Template Separator\n(You can make a copy of, or modify, this frame)"
        n358 = Unbundle By Name(w889) -> ("Preset Manager Cluster.My IP"=w888:string, "Preset Manager Cluster.PresetName"=w884:string)
        n359 = call "preset SQL Queries.vi"("Expt name / MCIP/ Variable/Preset Name"=w884, "Preset Query"=Preset_Query_Enum."GetPresetDeviceNames") -> ("1st column 1st data"=w886:string[])  [unwired: 7 in, 2 out]
        n360 = Concatenate Strings("preset>>" ("string"), w884, ">>" ("string"), w888) -> (w887:string)
        n361 = Bundle By Name(cluster=w889, "Preset Manager Cluster.PresetName"=w884, "Preset Manager Cluster.Mcast command"=w887, "Preset Manager Cluster.Current Preset Devices"=w886) -> (w890:T7)
        n362 = property on="Poll Count" class="DigNum (strict)"("Value"=0) -> ()  [unwired: 2 in, 2 out]
        n363 = call <vilib>:"Add State(s) to Queue__jki_lib_state_machine.vi"("State(s) in (\"\")"=w896, "State(s) at Back (\"\")"="Send Multicast>>Empty\nGeneral wait>>10\nSend Multicast>>Empty\nGeneral wait>>40\nSend Multicast\nGeneral wait>>500\nPoll Devices" ("Remaining States")) -> ("States Out"=w895:string)  [unwired: 13 in]
      }
      frame "Send Multicast" {
        w899 = "Empty" ("y")
        # "Template Separator\n(You can make a copy of, or modify, this frame)"
        n364 = Unbundle By Name(w904) -> ("Preset Manager Cluster.MCast Remote"=w909:u16, "Preset Manager Cluster.Mcast address"=w908:string, "Preset Manager Cluster.UDP timeout ms"=w906:i32, "Preset Manager Cluster.Mcast command"=w898:string, "Preset Manager Cluster.MC Multicast"=w905:refnum<k16>)
        n365 = Equal?(x=w901, y=w899) -> (x = y?=w900:bool)
        n366 = Select(t=w899, s=w900, f=w898) -> (s? t:f=w897:string)
        n367 = String To IP(1:w908) -> (0:w907:u32)
        n368 = UDP Write(address=w907, port or service name=w909, connection ID=w905, data in=w897, 9:w906) -> (3:w902:refnum<k16>)  [unwired: 1 in, 1 out]
        n369 = Bundle By Name(cluster=w904, "Preset Manager Cluster.MC Multicast"=w902) -> (w903:T7)
        n370 = call <vilib>:"Add State(s) to Queue__jki_lib_state_machine.vi"("State(s) in (\"\")"=w912) -> ("States Out"=w911:string)  [unwired: 14 in]
      }
      frame "-------------Diagnostics-----------" {
        # "Template Separator\n(You can make a copy of, or modify, this frame)"
        n371 = call <vilib>:"Add State(s) to Queue__jki_lib_state_machine.vi"("State(s) in (\"\")"=w916) -> ("States Out"=w915:string)  [unwired: 14 in]
      }
      frame "Execute Device Check" {
        # "Template Separator\n(You can make a copy of, or modify, this frame)"
        n372 = disable-structure shown="Enabled" {
          disable-tunnel: w918 -> [w924 _]
          disable-tunnel: [w923 _] -> w917
          frame Enabled {
            n373 = property on="Preset Devices Not On" class="LstBox (strict)"() -> ("Item Names"=w925:string[])  [unwired: 2 in, 2 out]
            n374 = property on="Preset Devices Not in Experiment" class="LstBox (strict)"() -> ("Item Names"=w926:string[])  [unwired: 2 in, 2 out]
            n375 = call-poly <userlib>:"Empty Array__ogtk.vi"("Array"=w925) -> ("Empty Array?"=w928:bool)  [unwired: 8 in]
            n376 = call-poly <userlib>:"Empty Array__ogtk.vi"("Array"=w926) -> ("Empty Array?"=w929:bool)  [unwired: 8 in]
            n377 = And(x=w929, y=w928) -> (x .and. y?=w927:bool)
            n378 = case shown="False" w927 {
              tunnel: [w930 w942] -> w923
              tunnel: w924 -> [w931 w942]
              frame False {
                n379 = Two Button Dialog(message="There are either some presets that are not in the \nexperiment or some devices are not on. Please\nif that would impact the preset excution. ", 1:"Stop Execution" ("F button name (\"Cancel\")"), 2:"Continue Execution" ("T button name (\"OK\")")) -> (T button?=w935:bool)
                n380 = case shown="True" w935 {
                  tunnel: ["" ("State(s) in Front (\"\")") w941] -> w930
                  tunnel: w931 -> [_ w941]
                  frame False {
                    w936 = FALSE
                    n381 = control-ref of="Preset Execution Indicator"() -> (w939:refnum<vi>)
                    n382 = property on="Queue Size" class="DigNum (strict)"("Visible"=w936) -> ()  [unwired: 2 in, 2 out]
                    n383 = property on="Current Preset Queue Element" class="Str"("Visible"=w936) -> ()  [unwired: 2 in, 2 out]
                    n384 = property on="Queue Progress Bar" class="Slide (strict)"("Visible"=w936) -> ()  [unwired: 2 in, 2 out]
                    n385 = property on="Property Node" class="Bool (strict)"(reference=w939, "Blinking"=FALSE, "Caption.Text"="" ("Boolean Text.Text")) -> ()  [unwired: 1 in, 2 out]
                  }
                  frame True {
                  }
                }
              }
              frame True {
              }
            }
          }
          frame Disabled {
          }
        }
        n386 = call <vilib>:"Add State(s) to Queue__jki_lib_state_machine.vi"("State(s) in Front (\"\")"=w917, "State(s) in (\"\")"=w922) -> ("States Out"=w921:string)  [unwired: 13 in]
      }
      frame "Expt Device Check" {
        # "Template Separator\n(You can make a copy of, or modify, this frame)"
        n387 = flat-sequence {
          tunnel: w944 -> [w963]
          tunnel: w943 -> [w958]
          frame #0 {
            n388 = call <vilib>:"Set Busy.vi"("disable click? (T)"=TRUE, "cursor ID"=refnum<k1> refnum) -> ()  [unwired: 8 in, 2 out]
          }
          frame #1 {
            n389 = Equal?(x=w958, y="Preset Only") -> (x = y?=w957:bool)
            n390 = case shown="True" w957 {
              tunnel: [enum16{"Preset Queue", "Preset Only"}."Preset Queue" ("Input Type") enum16{"Preset Queue", "Preset Only"}."Preset Only" ("Input Type")] -> w956
              frame False {
              }
              frame True {
              }
            }
            n391 = Unbundle By Name(w963) -> ("Preset Table Control"=w950:string[][], "Preset Manager Cluster.Experiment Name"=w954:string, "Preset Manager Cluster.PresetName"=w962:string, "Preset Manager Cluster.All Devices Core Info"=w953:string[][], "Preset Manager Cluster.DevStatusQueue"=w952:refnum<queue>)
            n392 = property on="Queue Table" class="Tbl (strict)"() -> ("Value"=w955:string[][])  [unwired: 2 in, 2 out]
            n393 = call "Devices Not On.vi"("All Devices Core Info"=w953, "Experiment"=w954, "Preset Table Control"=w950, "queue"=w952) -> ("Preset Devices Not Alive"=w951:string[])  [unwired: 6 in, 1 out]
            n394 = call "Preset Expt Device Comparison.vi"("Input Type"=w956, "Preset Name"=w962, "Preset Array"=w955, "Expt name"=w954) -> ("Devices Not in Experiment"=w960:string[], "Devices accounted for?"=w961:bool)  [unwired: 6 in]
            n395 = case shown="True" w961 {
              frame False {
                n396 = property on="Preset Execution Indicator" class="Bool (strict)"("Blinking"=FALSE, "Caption.Text"="Devices Not \nin Experiment" ("Boolean Text.Text"), "Value"=FALSE ("Blinking"), "Colors [4]"=cluster{u32, u32}[] [{16711680, 0}]) -> ()  [unwired: 2 in, 2 out]
              }
              frame True {
                n397 = property on="Preset Execution Indicator" class="Bool (strict)"("Blinking"=FALSE, "Caption.Text"="" ("Boolean Text.Text"), "Value"=FALSE ("Blinking"), "Colors [4]"=cluster{u32, u32}[] [{32639, 0}]) -> ()  [unwired: 2 in, 2 out]
              }
            }
            n398 = property on="Preset Devices Not in Experiment" class="LstBox (strict)"("Item Names"=w960) -> ()  [unwired: 2 in, 2 out]
            n399 = property on="Preset Devices Not On" class="LstBox (strict)"("Item Names"=w951) -> ()  [unwired: 2 in, 2 out]
          }
          frame #2 {
            n400 = call <vilib>:"Unset Busy.vi"() -> ()  [unwired: 11 in, 1 out]
          }
        }
        n401 = call <vilib>:"Add State(s) to Queue__jki_lib_state_machine.vi"("State(s) in (\"\")"=w947) -> ("States Out"=w946:string)  [unwired: 14 in]
      }
      frame "Check Expt Device On" {
        # "Template Separator\n(You can make a copy of, or modify, this frame)"
        n402 = Unbundle By Name(w979) -> ("Preset Manager Cluster.Experiment Name"=w978:string, "Preset Manager Cluster.All Devices Core Info"=w977:string[][], "Preset Manager Cluster.DevStatusQueue"=w976:refnum<queue>, "Preset Table Control"=w974:string[][])  [unwired: 1 out]
        n403 = call "Devices Not On.vi"("All Devices Core Info"=w977, "Experiment"=w978, "Preset Table Control"=w974, "queue"=w976) -> ("Preset Devices Not Alive"=w975:string[])  [unwired: 6 in, 1 out]
        n404 = property on="Preset Devices Not On" class="LstBox (strict)"("Item Names"=w975) -> ()  [unwired: 2 in, 2 out]
        n405 = call <vilib>:"Add State(s) to Queue__jki_lib_state_machine.vi"("State(s) in (\"\")"=w982) -> ("States Out"=w981:string)  [unwired: 14 in]
      }
    }
  }
  "Currently Loaded" <- ""
